vi "All-In-One_EIC-DIRC_DAQ_v2-1.vi"() -> ()   [LabVIEW 2024]
uses:
  C:/Users/hpDIRC/Desktop/eic_dirc_daq-LabVIEW_new/Thorlabs.MotionControl.Controls.dll
  Thorlabs.MotionControl.Controls.dll
  <vilib>/numeric/Random Number (Range) DBL.vi
  C:/Users/hpDIRC/Desktop/eic_dirc_daq-LabVIEW_new/Thorlabs.MotionControl.IntegratedStepperMotorsCLI.dll
  Thorlabs.MotionControl.IntegratedStepperMotorsCLI.dll
  C:/Users/hpDIRC/Desktop/eic_dirc_daq-LabVIEW_new/Thorlabs.MotionControl.Benchtop.StepperMotorCLI.dll
  Thorlabs.MotionControl.Benchtop.StepperMotorCLI.dll
  <instrlib>/Keithley 6517/Keithley 6517.lvlib
panel:
  out "NM-pts-tested":dbl caption="# Pts Tested for Alignment"
  in  "align-only":bool
  in  "run-BA":bool
  in  "run-IR":bool
  in  "PDY start":dbl=105.8
  in  "PDX start":dbl=265.0
  out "run time (min)":dbl
  out "alignment-counter":dbl=184.0 format="%#_13g"
  out "Optimized Location":dbl[](array[numeric])
  in  "Test Start Delay (s)":dbl=30.0
  out "queue-length":i32 caption="Queue Elements Remaining:"
  out "next-state-cluster-const":T1={"next-state"="", "bypass-confirm"=FALSE, "PDX"=300.0, "PDY"=150.0, "BarX"=300.0, "BarY"=150.0, "BMA"=45.0, "PDA"=85.0, "bar-note"=0, "meas#"=0}
  in  "X start":dbl=262.0
  in  "X end":dbl=263.0
  in  "Y end":dbl=121.5 format="%#_13g"
  in  "X step size":dbl=0.2 format="%#_13g"
  in  "Y step size":dbl=0.2
  in  "Y start":dbl=120.5 format="%#_13g"
  in  "centered-diode-scan":bool
  out "keep-file":bool
  out "status":string
  out "queue-size":i32
  in  "save-loc":bool
  out "stored-pos":T2 caption="Location Stored"
  out "main-stage-refs":T3
  out "state-queue":T4(array[cluster])
  in  "PDA":dbl=184.0 format="%#_13g"
  in  "BMA":dbl=45.0 format="%#_13g"
  in  "BarY":dbl=30.0 format="%#_13g"
  in  "BarX":dbl=230.0 format="%#_13g"
  in  "PDY":dbl=124.0 format="%#_13g"
  in  "PDX":dbl=274.0 format="%#_13g"
  out "bypass-confirm":bool
  out "PD Values":cluster{"PD1":dbl, "PD2":dbl, "PD3":dbl}
  out "last-PD":dbl[](array[numeric])=[1.0, 1.0, 1.0]
  in  "move-bar":bool
  out "pd_angle":dbl
  out "brewster_angle":dbl
  out "meter-visa":refnum<visa-resource-name>
  out "loop-rate":u32
  out "meter-stat":bool caption="Log Status"
  out "file-stat":bool caption="Log Status"
  out "stage-stat":bool caption="Log Status"
  out "last-save-time":string caption="Time of Last Save:"
  out "pd_y_pos":dbl
  out "pd_x_pos":dbl
  out "bar_y_pos":dbl
  out "bar_x_pos":dbl
  in  "nSamples":dbl=50.0 caption="# Samples"
  out "Current Time:":string
  in  "save-data":bool
  in  "bar-note":u16(ring) items=["Pure Beam (PB)", "Internal Reflection (IR)", "Bulk Attenuation (BA)"]
  out "pd3_v":dbl caption="PD 3" format="%#.4g"
  out "pd2_v":dbl caption="PD 2" format="%#.4g"
  out "pd1_v":dbl caption="PD 1" format="%#.4g"
  out "meter-error":errorcluster
  out "log-error":errorcluster
  out "log-path":path caption="Path Data Will Save To:"
  out "start-msg":string
  out "stage-error":errorcluster
  in  "PD Angle":refnum<k24>(container)
  in  "Brewster":refnum<k24>(container)
  in  "PD Y":refnum<k24>(container)
  in  "PD X":refnum<k24>(container)
  in  "BAR Y":refnum<k24>(container)
  in  "stop":bool
  in  "BAR X":refnum<k24>(container)
  out "pd-plt":cluster{"[0]":dbl, "[1]":dbl, "[2]":dbl}(graph) caption="Measurement History"
  # "EXPERT DEBUGGING INFO"
  # "A"
  # "A"
  # "A"
  # "Work In Progress - please do not use"
  # "Bar Note Readback:"
  # "PD ONLY SCAN - CENTERED"
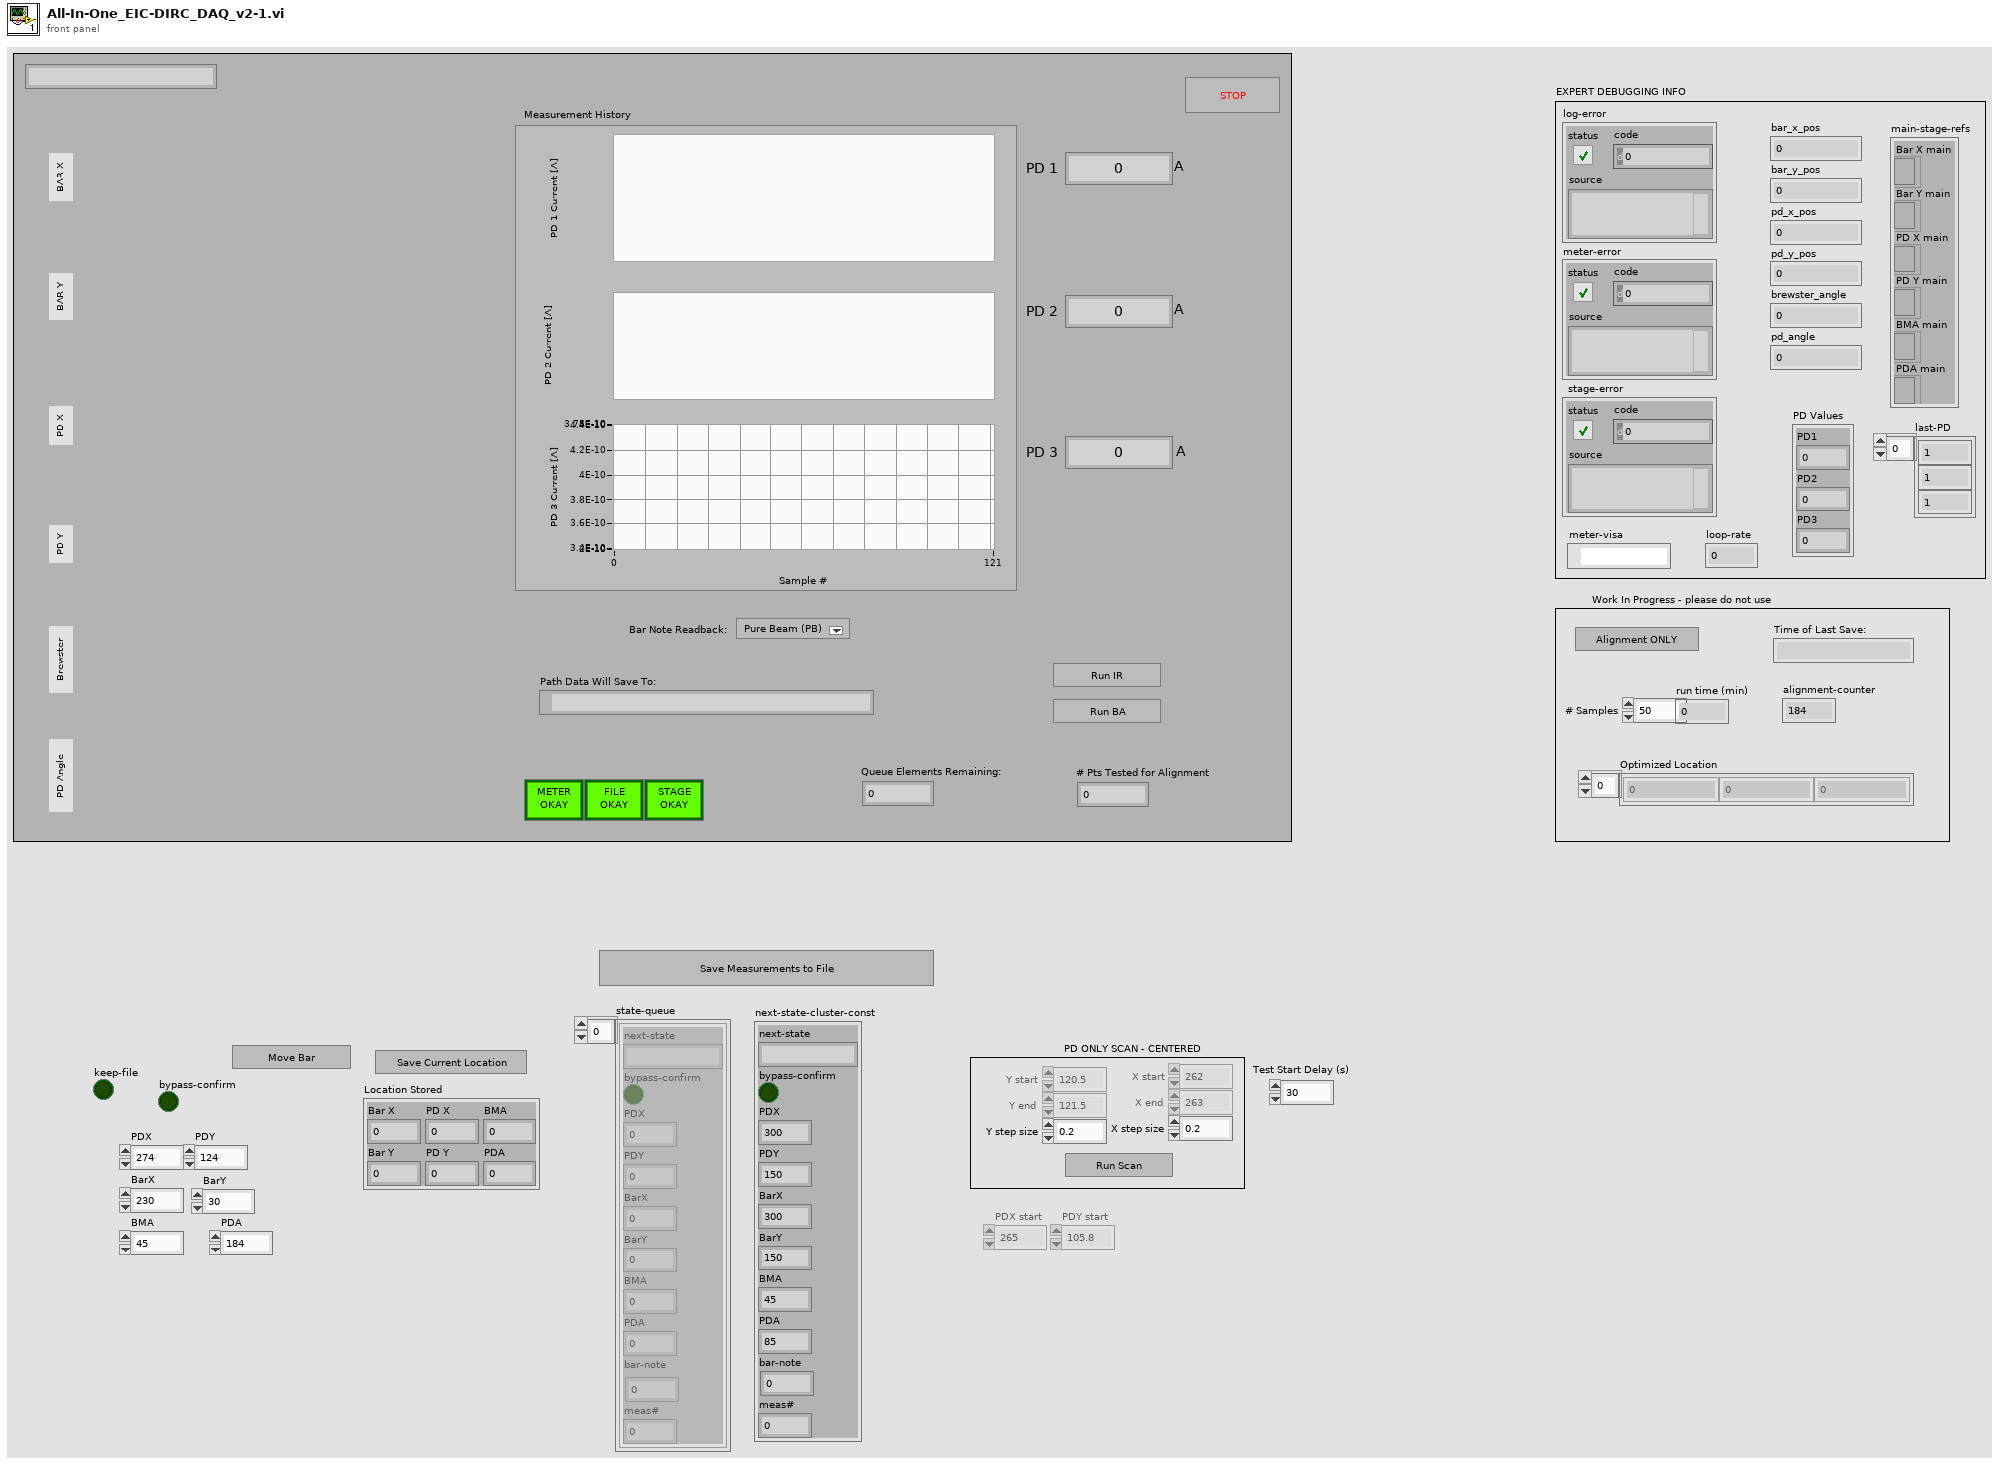
[diagram p1: front panel]
types:
  T1 = cluster{"next-state":string, "bypass-confirm":bool, "PDX":dbl, "PDY":dbl, "BarX":dbl, "BarY":dbl, "BMA":dbl, "PDA":dbl, "bar-note":u8, "meas#":u32}
  T2 = cluster{"Bar X":dbl, "Bar Y":dbl, "PD X":dbl, "PD Y":dbl, "BMA":dbl, "PDA":dbl}
  T3 = cluster{"Bar X main":refnum<k24>, "Bar Y main":refnum<k24>, "PD X main":refnum<k24>, "PD Y main":refnum<k24>, "BMA main":refnum<k24>, "PDA main":refnum<k24>}
  T4 = cluster{"next-state":string, "bypass-confirm":bool, "PDX":dbl, "PDY":dbl, "BarX":dbl, "BarY":dbl, "BMA":dbl, "PDA":dbl, "bar-note":u8, "meas#":u32}[]
  T5 = cluster{"Bar X":refnum<k24>, "Bar Y":refnum<k24>, "PD X":refnum<k24>, "PD Y":refnum<k24>, "Brewster":refnum<k24>, "PD Angle":refnum<k24>}
  T6 = enum16{"open", "replace", "create", "open or create", "replace or create", "replace or create with confirmation"}
  T7 = cluster{"alpha":dbl, "gamma":dbl, "rho":dbl, "sigma":dbl, "simplex L":dbl}
  T8 = cluster{"next-state":string, "mode-select":enum32{"IR", "Pure", "Bulk", "Bar Out", "stored-loc", "custom"}, "bypass-confirm":bool, "PDX":dbl, "PDY":dbl, "BarX":dbl, "BarY":dbl, "BMA":dbl, "PDA":dbl, "bar-note":bool}
  T9 = cluster{"error":bool, "code":i32, "source":string}
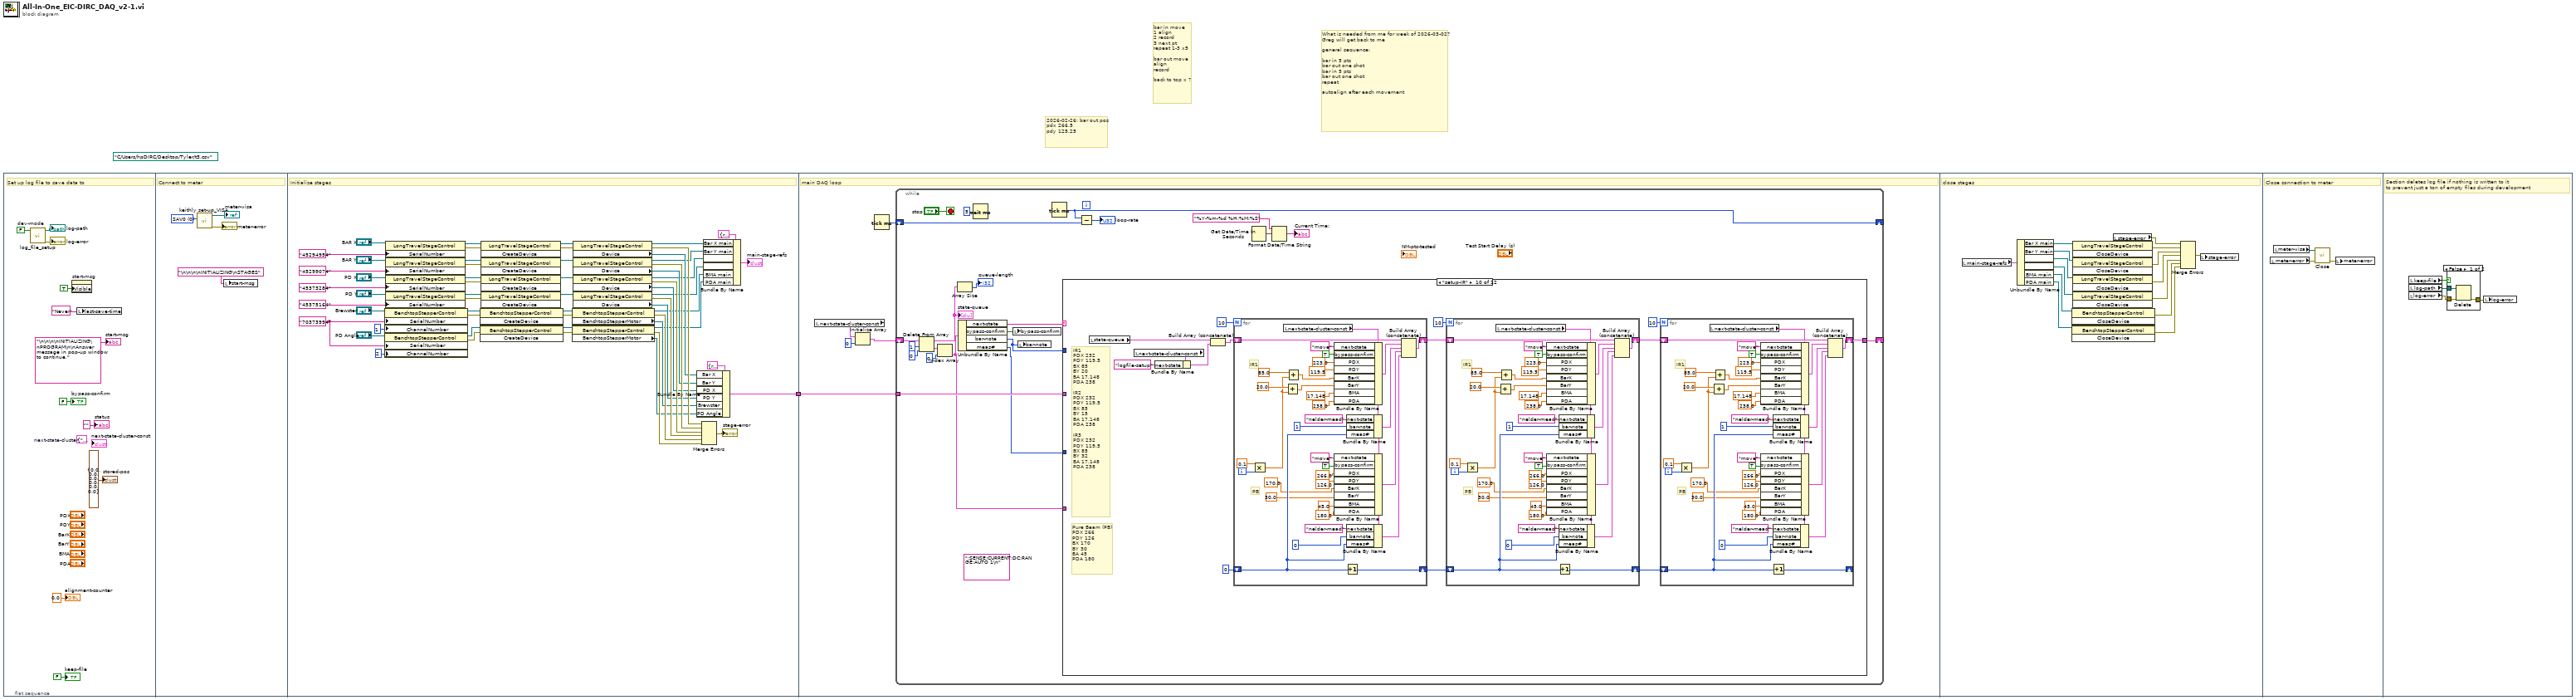
[diagram p0: block diagram]
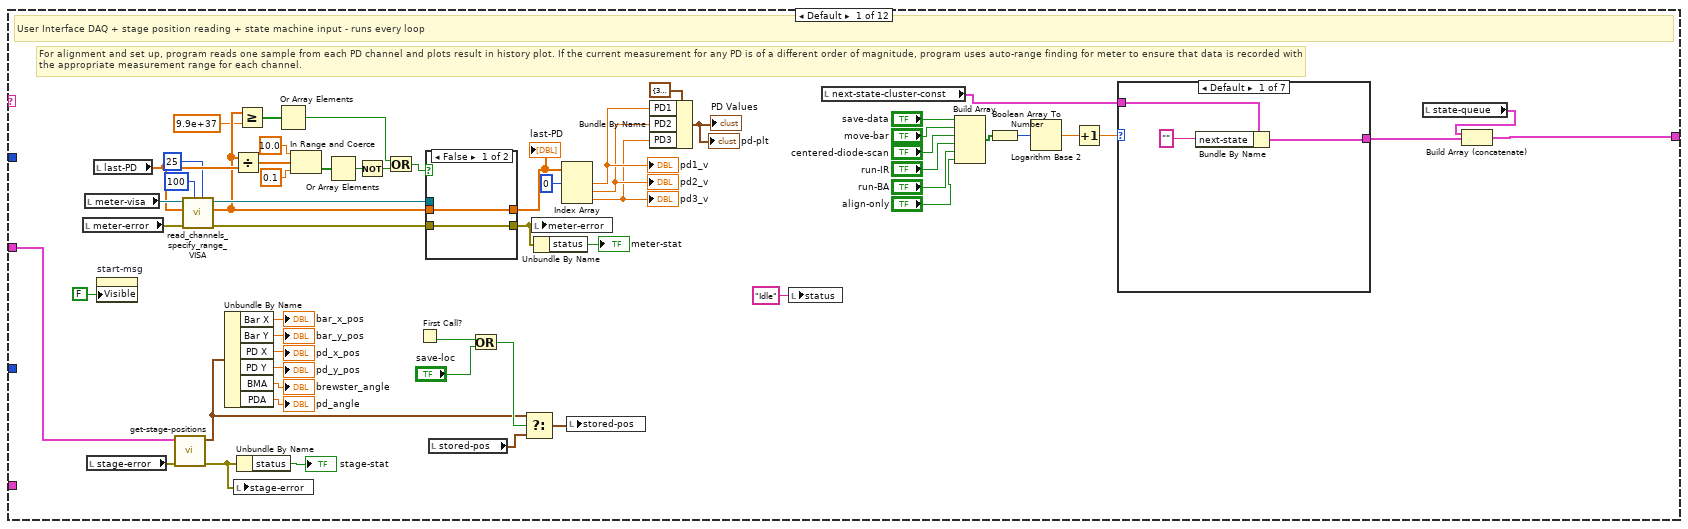
[diagram p2: hidden frame]
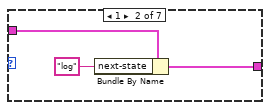
[diagram p3: hidden frame]
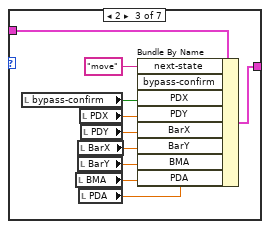
[diagram p4: hidden frame]
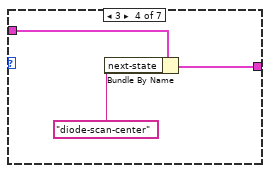
[diagram p5: hidden frame]
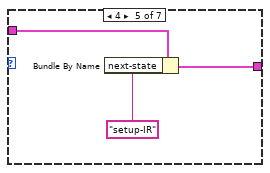
[diagram p6: hidden frame]
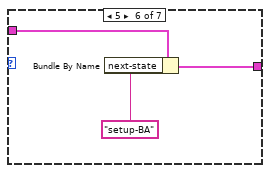
[diagram p7: hidden frame]
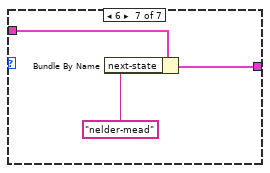
[diagram p8: hidden frame]
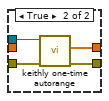
[diagram p9: hidden frame]
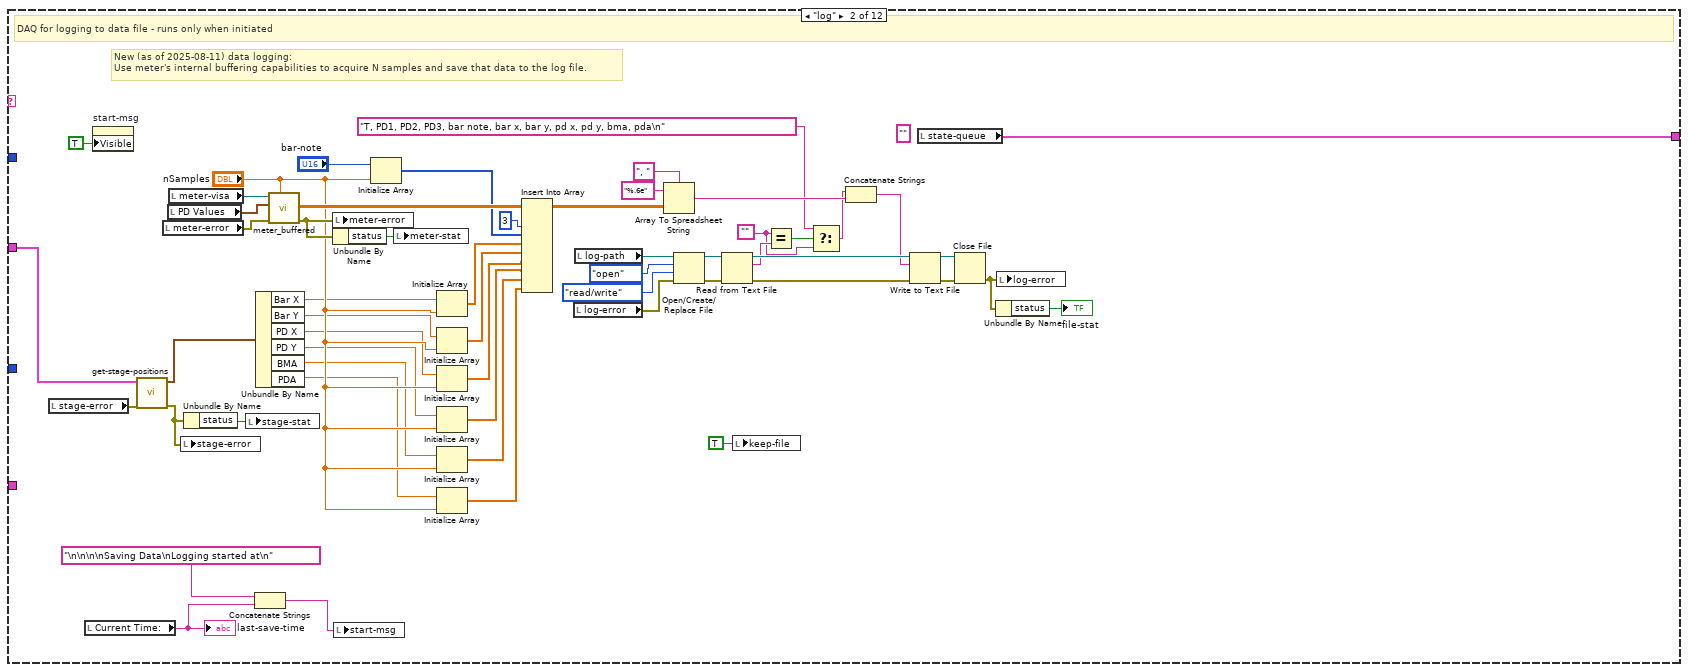
[diagram p10: hidden frame]
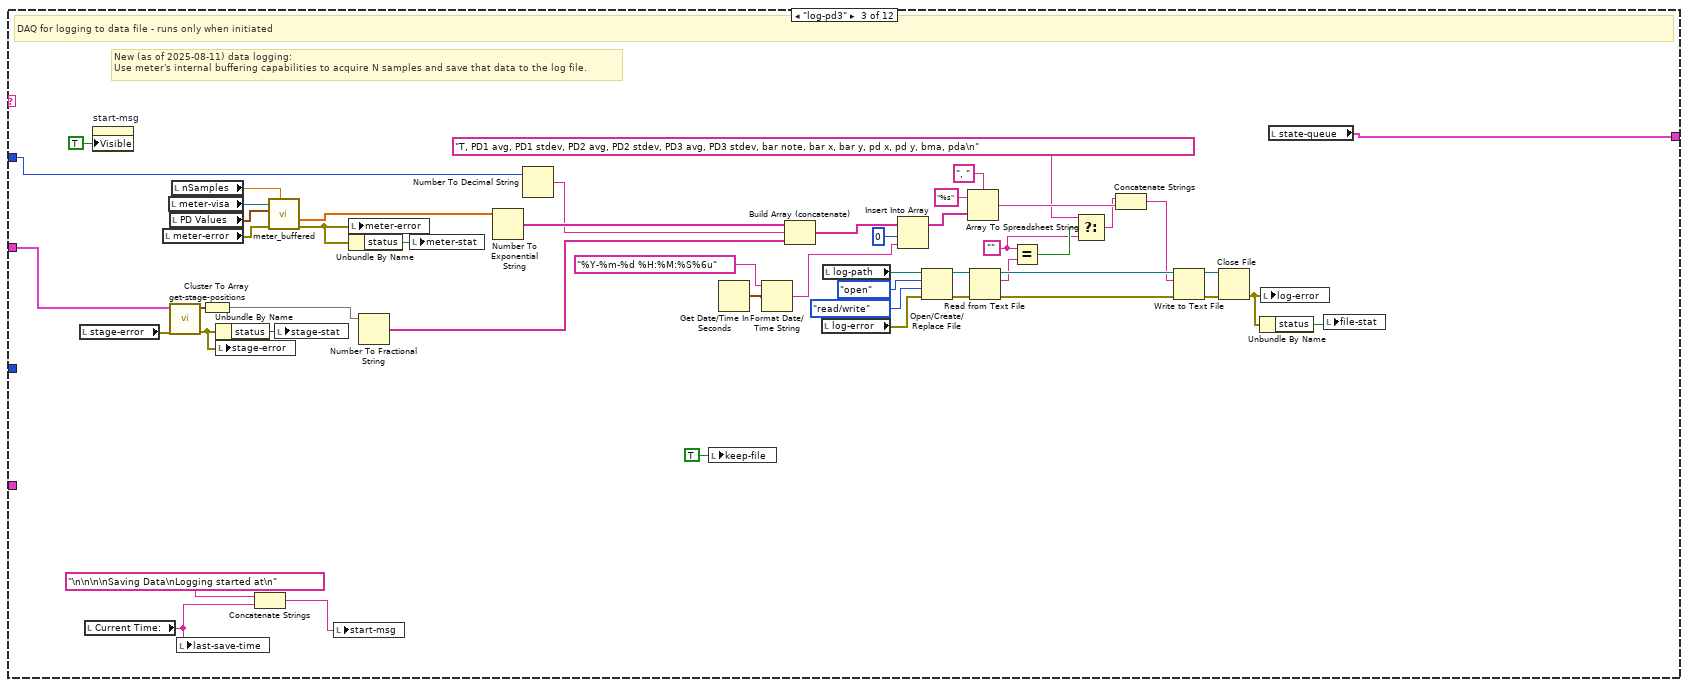
[diagram p11: hidden frame]
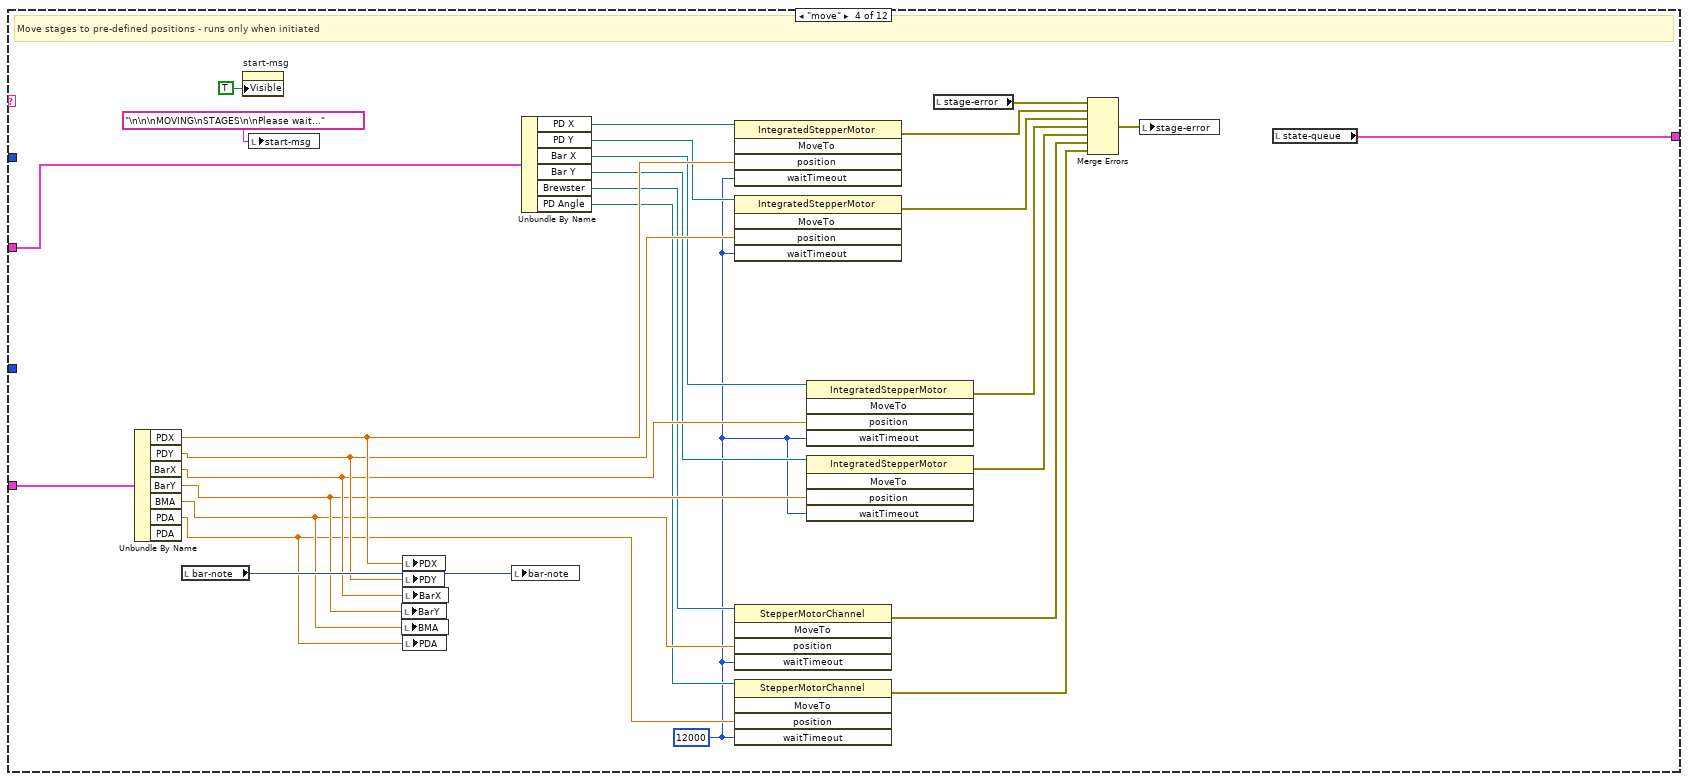
[diagram p12: hidden frame]
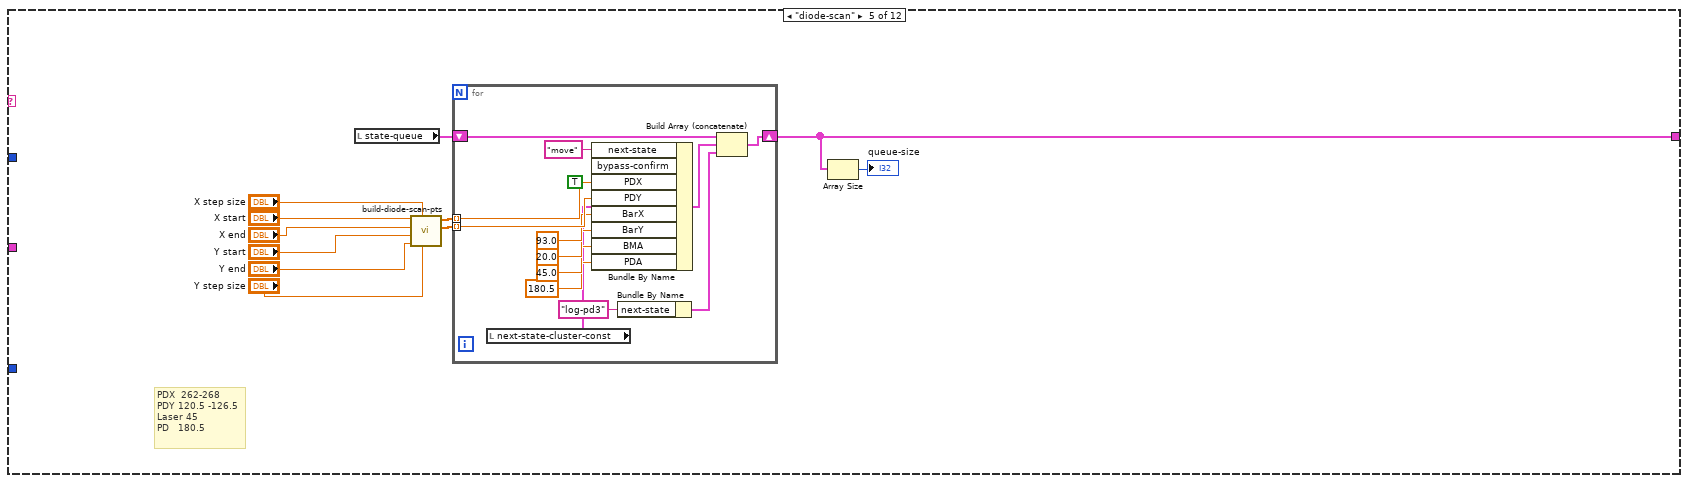
[diagram p13: hidden frame]
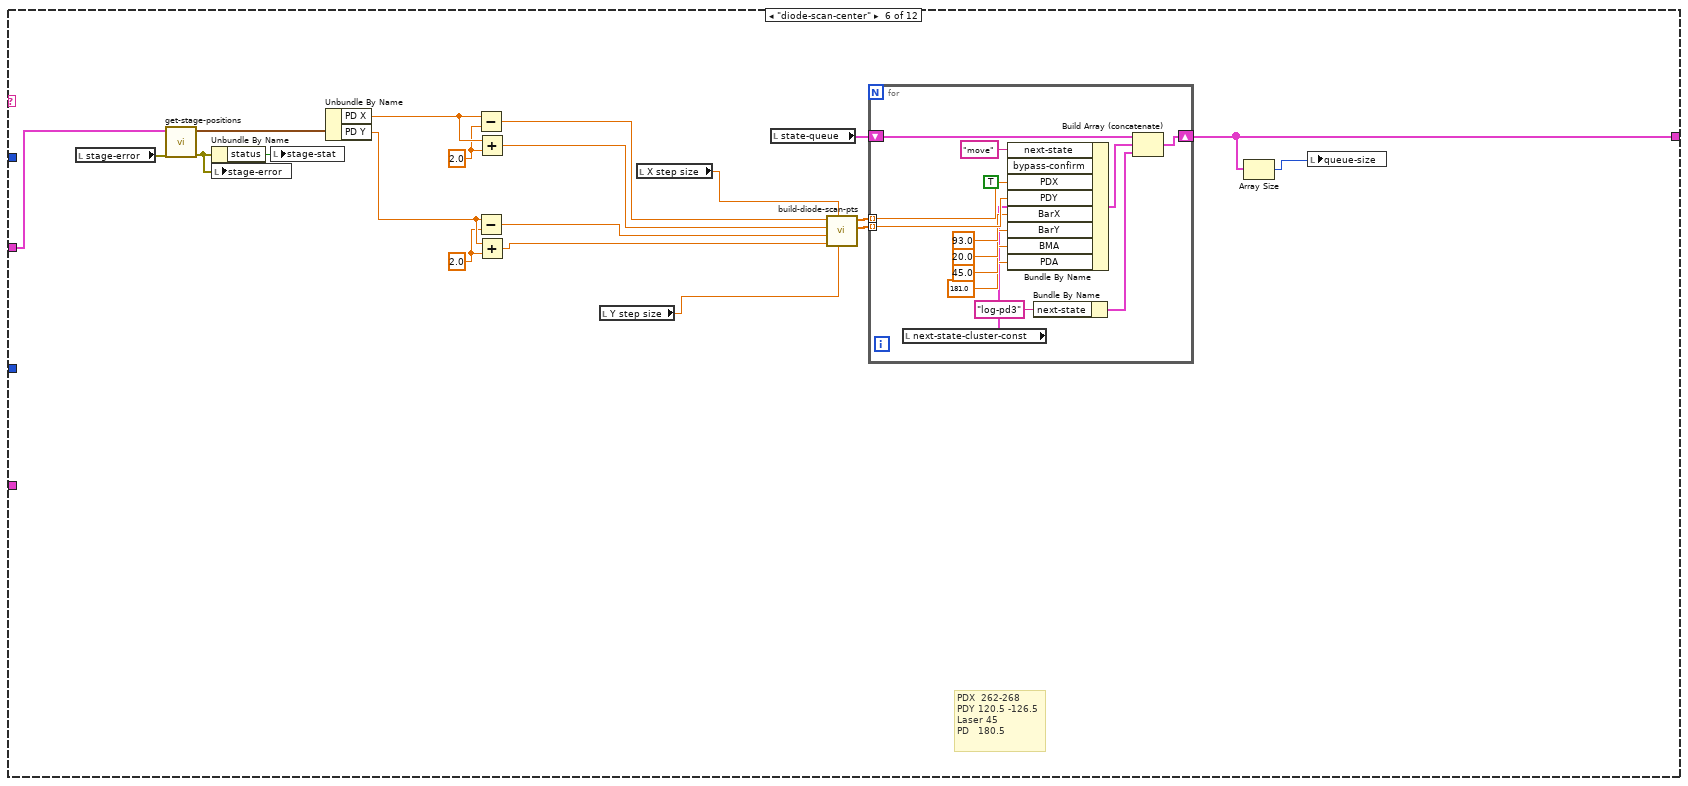
[diagram p14: hidden frame]
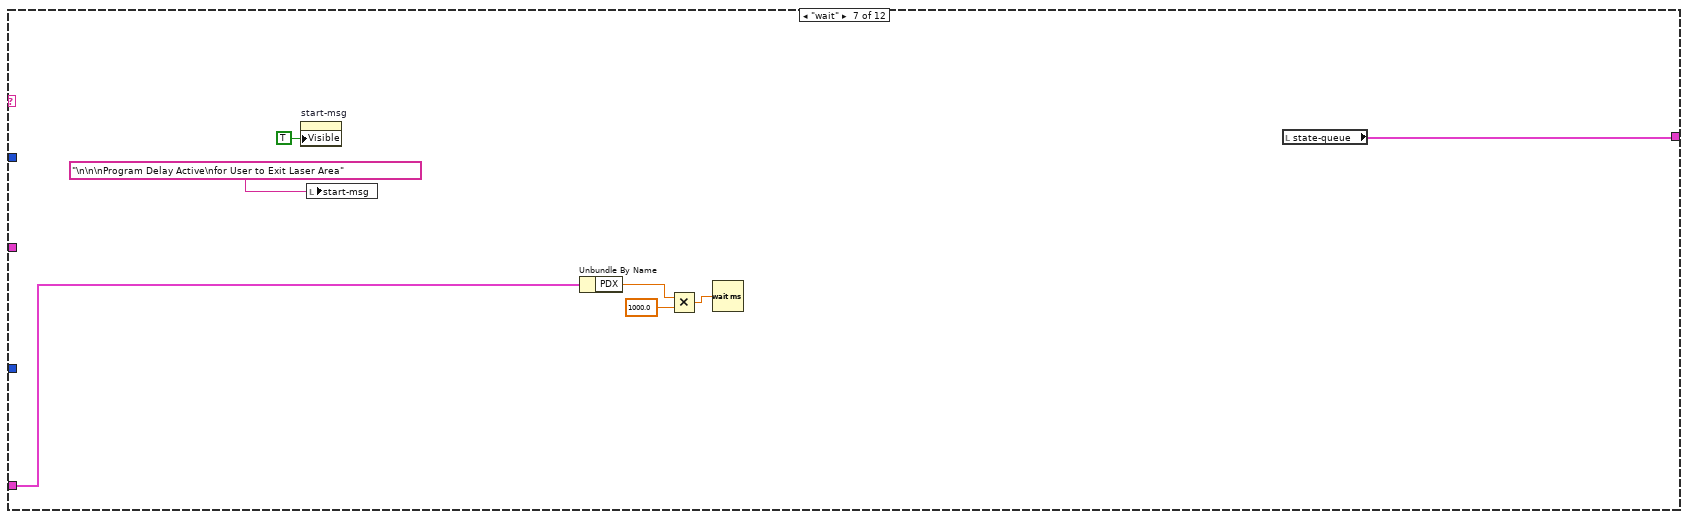
[diagram p15: hidden frame]
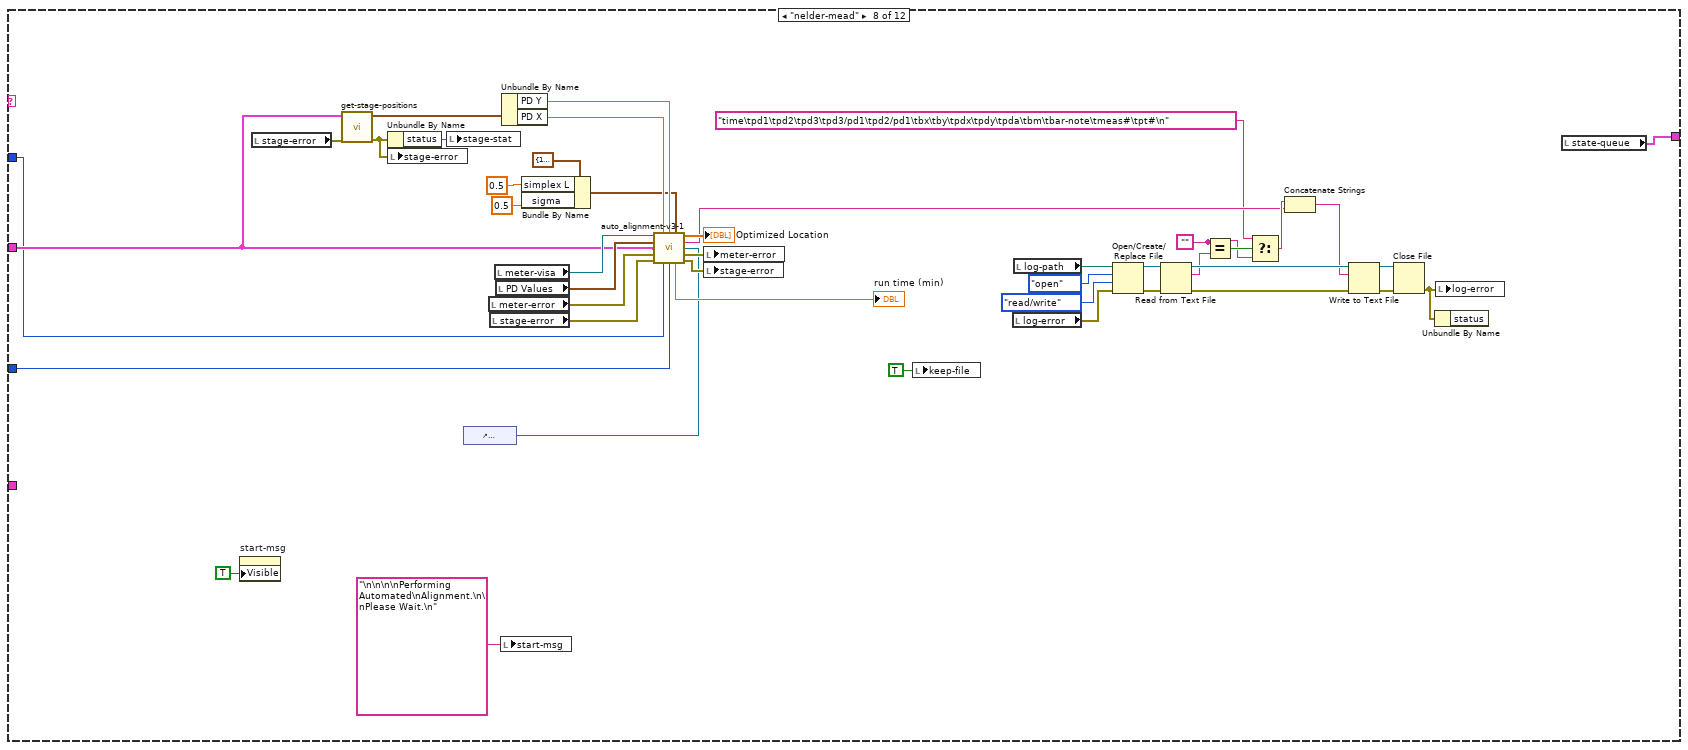
[diagram p16: hidden frame]
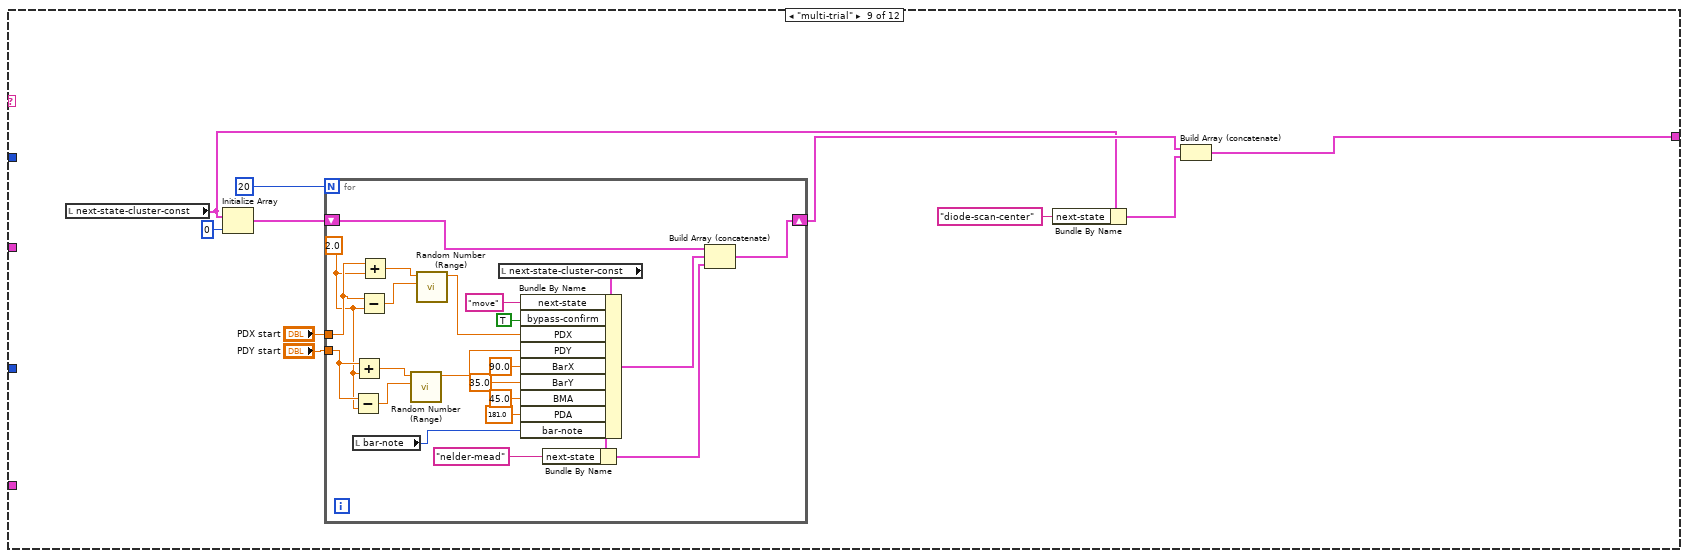
[diagram p17: hidden frame]
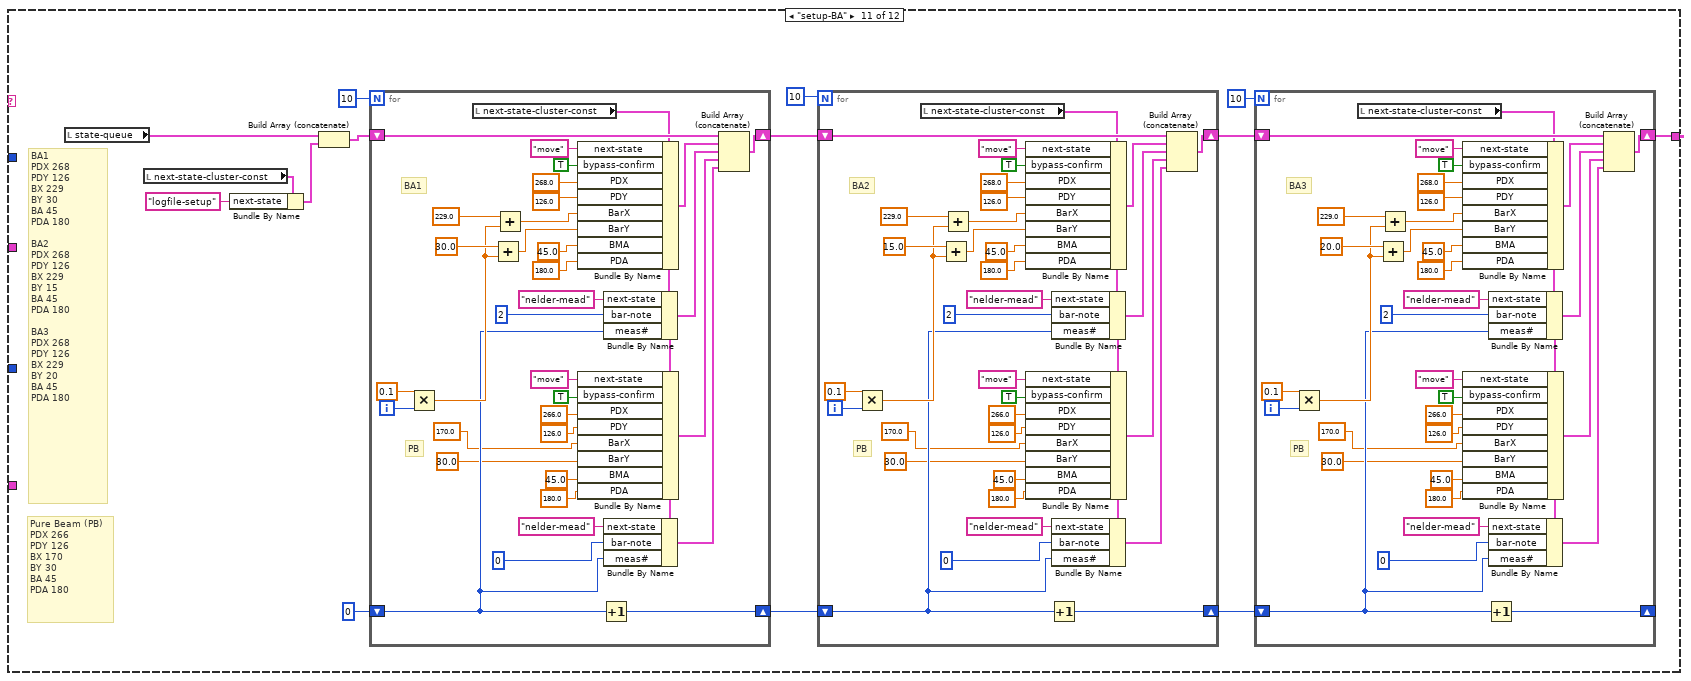
[diagram p18: hidden frame]
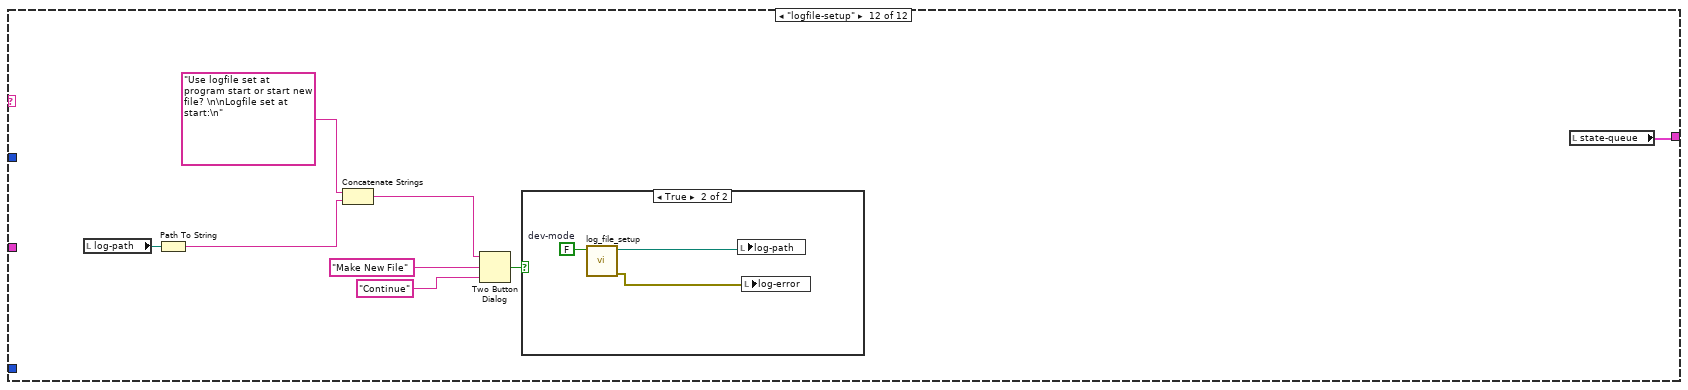
[diagram p19: hidden frame]
diagram:
  (unwired) path "C:/Users/hpDIRC/Desktop/Tyler/t3.csv" ("log-path")
  # "2026-02-26: bar out pos\npdx 266.5\npdy 125.25"
  # "bar in move\n1 align\n2 record\n3 next pt\nrepeat 1-3 x5\n\nbar out move\nalign\nrecord\n\nback to top x ?"
  # "What is needed from me for week of 2026-03-02?\nGreg will get back to me\n\ngeneral sequence:\n\nbar in 5 pts \nbar out one shot\nbar in 5 pts\nbar out one shot\nrepeat\n\nautoalign after each movement"
  n1 = flat-sequence {
    tunnel: [w25] -> w1
    tunnel: w1 -> [w77]
    frame #0 {
      w4 = FALSE  # dev-mode
      (unwired) T8 {"next-state"="", "mode-select"=enum."IR", "bypass-confirm"=FALSE, "PDX"=300.0, "PDY"=150.0, "BarX"=300.0, "BarY"=150.0, "BMA"=45.0, "PDA"=85.0, "bar-note"=FALSE}  # next-state-cluster
      # "Set up log file to save data to"
      n2 = call "log_file_setup.vi"("dev-mode"=w4) -> ("error out"=→"log-error":errorcluster, "appended path"=→"log-path":path)  [unwired: 8 in, 1 out]
      n3 = property on="start-msg" class="Str"("Visible"=TRUE) -> ()  [unwired: 2 in, 2 out]
      n4 = local write "last-save-time"("Never" ("date/time string")) -> ()
      "start-msg" <- "\n\n\n\nINITIALIZING\nPROGRAM\n\nAnswer message in pop-up window to continue." ("String")
      "bypass-confirm" <- FALSE
      "stored-pos" <- T2 {"Bar X"=0.0, "Bar Y"=0.0, "PD X"=0.0, "PD Y"=0.0, "BMA"=0.0, "PDA"=0.0} ("stage-pos")
      "status" <- "" ("status")
      "keep-file" <- FALSE
      "alignment-counter" <- 0.0 ("alignment-counter")
    }
    frame #1 {
      w13 = i16 0 items=["SAV0", "SAV1", "SAV2", "SAV3", "SAV4", "SAV5", "SAV6", "SAV7", "SAV8", "SAV9", "RST", "Preset"] ("ConfigOpt")
      # "Connect to meter"
      n5 = call "keithly set-up_VISA.vi"("ConfigOpt"=w13) -> ("error out"=→"meter-error":errorcluster, "meter-VISA"=→"meter-visa":refnum<visa-resource-name>)  [unwired: 9 in]
      n6 = local write "start-msg"("\n\n\n\nINITIALIZING\nSTAGES" ("String")) -> ()
    }
    frame #2 {
      w32 = "70373994" ("SerialNumber")
      # "Initialize stages"
      n7 = property class="BenchtopStepperControl"(reference="Brewster", "SerialNumber"=w32, "ChannelNumber"=1) -> (reference out=w58:refnum<k24>, error out=w59:errorcluster)  [unwired: 1 in]
      n8 = property class="BenchtopStepperControl"(reference="PD Angle", "SerialNumber"=w32, "ChannelNumber"=2) -> (reference out=w57:refnum<k24>, error out=w60:errorcluster)  [unwired: 1 in]
      n9 = property class="LongTravelStageControl"(reference="BAR X", "SerialNumber"="45294954") -> (reference out=w35:refnum<k24>, error out=w42:errorcluster)  [unwired: 1 in]
      n10 = property class="LongTravelStageControl"(reference="BAR Y", "SerialNumber"="45299074") -> (reference out=w36:refnum<k24>, error out=w43:errorcluster)  [unwired: 1 in]
      n11 = property class="LongTravelStageControl"(reference="PD X", "SerialNumber"="45373284") -> (reference out=w39:refnum<k24>, error out=w44:errorcluster)  [unwired: 1 in]
      n12 = property class="LongTravelStageControl"(reference="PD Y", "SerialNumber"="45375164") -> (reference out=w40:refnum<k24>, error out=w45:errorcluster)  [unwired: 1 in]
      n13 = invoke class="BenchtopStepperControl" method="CreateDevice"(reference=w58, error in=w59) -> (reference out=w55:refnum<k24>, error out=w53:errorcluster)  [unwired: 1 in, 1 out]
      n14 = invoke class="BenchtopStepperControl" method="CreateDevice"(reference=w57, error in=w60) -> (reference out=w54:refnum<k24>, error out=w56:errorcluster)  [unwired: 1 in, 1 out]
      n15 = invoke class="LongTravelStageControl" method="CreateDevice"(reference=w35, error in=w42) -> (reference out=w48:refnum<k24>, error out=w52:errorcluster)  [unwired: 1 in, 1 out]
      n16 = invoke class="LongTravelStageControl" method="CreateDevice"(reference=w36, error in=w43) -> (reference out=w49:refnum<k24>)  [unwired: 1 in, 2 out]
      n17 = invoke class="LongTravelStageControl" method="CreateDevice"(reference=w39, error in=w44) -> (reference out=w50:refnum<k24>)  [unwired: 1 in, 2 out]
      n18 = invoke class="LongTravelStageControl" method="CreateDevice"(reference=w40, error in=w45) -> (reference out=w51:refnum<k24>)  [unwired: 1 in, 2 out]
      n19 = property class="BenchtopStepperControl"(reference=w55, error in=w53) -> (reference out=w19:refnum<k24>, error out=w70:errorcluster, "BenchtopStepperMotor"=w65:refnum<k24>)
      n20 = property class="BenchtopStepperControl"(reference=w54, error in=w56) -> (reference out=w18:refnum<k24>, error out=w71:errorcluster, "BenchtopStepperMotor"=w66:refnum<k24>)
      n21 = property class="LongTravelStageControl"(reference=w48, error in=w52) -> (reference out=w23:refnum<k24>, error out=w72:errorcluster, "Device"=w61:refnum<k24>)
      n22 = property class="LongTravelStageControl"(reference=w49) -> (reference out=w22:refnum<k24>, error out=w67:errorcluster, "Device"=w62:refnum<k24>)  [unwired: 1 in]
      n23 = property class="LongTravelStageControl"(reference=w50) -> (reference out=w21:refnum<k24>, error out=w68:errorcluster, "Device"=w63:refnum<k24>)  [unwired: 1 in]
      n24 = property class="LongTravelStageControl"(reference=w51) -> (reference out=w20:refnum<k24>, error out=w69:errorcluster, "Device"=w64:refnum<k24>)  [unwired: 1 in]
      n25 = Bundle By Name(cluster=T5 {"Bar X"=refnum, "Bar Y"=refnum, "PD X"=refnum, "PD Y"=refnum, "Brewster"=refnum, "PD Angle"=refnum}, "Bar X"=w61, "Bar Y"=w62, "PD X"=w63, "PD Y"=w64, "Brewster"=w65, "PD Angle"=w66) -> (w25:T5)
      n26 = Merge Errors(w72, w67, w68, w69, w70, w71) -> (→"stage-error":errorcluster)
      n27 = Bundle By Name(cluster=T3 {"Bar X main"=refnum, "Bar Y main"=refnum, "PD X main"=refnum, "PD Y main"=refnum, "BMA main"=refnum, "PDA main"=refnum}, "Bar X main"=w23, "Bar Y main"=w22, "PD X main"=w21, "PD Y main"=w20, "BMA main"=w19, "PDA main"=w18) -> (→"main-stage-refs":T3)
    }
    frame #3 {
      # "main DAQ loop"
      n28 = local read "next-state-cluster-const"() -> (w74:T1)
      n29 = Initialize Array(w74, 0 ("dimension size")) -> (w76:T4)
      n30 = Tick Count (ms)() -> (millisecond timer value=w78:u32)
      n31 = while {
        shift-right: [w99] -> _
        shift-left: w78 -> [w98]
        tunnel: w77 -> [w96]
        shift-right: [w84] -> _
        shift-left: w76 -> [w86]
        stop <- "stop" stop-if-true
        (unwired) ":SENSE:CURRENT:DC:RANGE:AUTO 1\n"
        n32 = Delete From Array(array=w86, length=1, index=0) -> (deleted portion=w85:T4, array with subset deleted=w82:T4)
        "state-queue" <- w82
        n33 = Index Array(array=w85, index=0) -> (element=w83:T1)
        n34 = Array Size(array=w82) -> (size(s)=→"queue-length":i32)
        n35 = Unbundle By Name(w83) -> ("next-state"=w88:string, "bypass-confirm"=w87:bool, "bar-note"=w81:u8, "meas#"=w80:u32)
        n36 = Wait (ms)(milliseconds to wait=u32 5) -> ()  [unwired: 1 out]
        n37 = local write "bypass-confirm"(w87) -> ()
        n38 = local write "bar-note"(w81) -> ()
        n39 = Tick Count (ms)() -> (millisecond timer value=w99:u32)
        n40 = case shown="\"setup-IR\"" w88 {
          tunnel: w96 -> [w151 w212 w277 w324 _ w359 _ w414 _ _ _ _]
          tunnel: [w123 w223 w282 w323 w333 w367 w387 w435 w438 w472 w588 w707] -> w84
          tunnel: w83 -> [_ _ _ w320 _ _ w388 _ _ _ _ _]
          tunnel: w81 -> [_ _ w260 _ _ _ _ w413 _ _ _ _]
          tunnel: w80 -> [_ _ _ _ _ _ _ w412 _ _ _ _]
          frame Default {
            # "For alignment and set up, program reads one sample from each PD channel and plots result in history plot. If the current measurement for any PD is of a different order of magnitude, program uses auto-range finding for meter to ensure that data is recorded with the appropriate measurement range for each channel."
            # "User Interface DAQ + stage position reading + state machine input - runs every loop"
            n41 = local read "meter-error"() -> (w148:errorcluster)
            n42 = local read "meter-visa"() -> (w149:refnum<visa-resource-name>)
            n43 = local read "stage-error"() -> (w150:errorcluster)
            n44 = local read "last-PD"() -> (w139:dbl[])
            n45 = property on="start-msg" class="Str"("Visible"=FALSE) -> ()  [unwired: 2 in, 2 out]
            n46 = call "get-stage-positions.vi"("error in (no error)"=w150, "Cluster"=w151) -> ("error out"=w136:errorcluster, "stage positions"=w109:T2)  [unwired: 8 in]
            n47 = call "read_channels_specify_range_VISA.vi"("postDAQ  wait ms"=u32 25, "preDAQ  wait ms"=u32 100, "error in"=w148, "range"=w139, "VISA resource in"=w149) -> ("error out"=w141:T9, "data"=w129:dbl[], "VISA resource out"=w140:refnum<visa-resource-name>)  [unwired: 4 in]
            n48 = Unbundle By Name(w109) -> ("Bar X"=→"bar_x_pos":dbl, "Bar Y"=→"bar_y_pos":dbl, "PD X"=→"pd_x_pos":dbl, "PD Y"=→"pd_y_pos":dbl, "BMA"=→"brewster_angle":dbl, "PDA"=→"pd_angle":dbl)
            n49 = Divide(x=w129, y=w139) -> (x/y=w144:dbl[])
            n50 = local write "stage-error"(w136) -> ()
            n51 = Greater Or Equal?(x=w129, y=9.9e+37) -> (x >= y?=w127:bool[])
            n52 = Unbundle By Name(w136) -> ("status"=→"stage-stat":bool)
            n53 = Or Array Elements(Boolean array=w127) -> (logical OR=w126:bool)
            n54 = In Range and Coerce(upper limit=10.0, x=w144, lower limit=0.1) -> (In Range?=w142:bool[])  [unwired: 1 out]
            n55 = Or Array Elements(Boolean array=w142) -> (logical OR=w143:bool)
            n56 = Not(x=w143) -> (.not. x?=w131:bool)
            n57 = Or(x=w126, y=w131) -> (x .or. y?=w130:bool)
            n58 = First Call?() -> (First Call?: T/F=w119:bool)
            n59 = case shown="False" w130 {
              tunnel: w141 -> [w189 w193]
              tunnel: [w189 w192] -> w157
              tunnel: [w188 w191] -> w152
              tunnel: w129 -> [w188 _]
              tunnel: w140 -> [_ w190]
              frame False {
              }
              frame True {
                n60 = call "keithly one-time autorange.vi"("error in"=w193, "VISA in"=w190) -> ("error out"=w192:errorcluster, "data"=w191:dbl[])  [unwired: 7 in, 1 out]
              }
            }
            "last-PD" <- w152
            n61 = local read "stored-pos"() -> (w120:T2)
            n62 = Or(x=w119, y="save-loc") -> (x .or. y?=w117:bool)
            n63 = Select(t=w109, s=w117, f=w120) -> (s? t:f=w121:T2)
            n64 = local write "meter-error"(w157) -> ()
            n65 = Unbundle By Name(w157) -> ("status"=→"meter-stat":bool)
            n66 = Index Array(array=w152, index #1=0 ("index")) -> (element #1=w155:dbl, element #2=w154:dbl, element #3=w153:dbl)  [unwired: 2 in]
            "pd3_v" <- w153
            "pd2_v" <- w154
            "pd1_v" <- w155
            n67 = local write "stored-pos"(w121) -> ()
            n68 = Bundle By Name(cluster=cluster{"PD1":dbl, "PD2":dbl, "PD3":dbl} {"PD1"=3e-05, "PD2"=3e-05, "PD3"=3e-05} ("PD ranges"), "PD1"=w155, "PD2"=w154, "PD3"=w153) -> (→"pd-plt" →"PD Values":cluster{"PD1":dbl, "PD2":dbl, "PD3":dbl})
            n69 = local write "status"("Idle" ("status")) -> ()
            n70 = local read "next-state-cluster-const"() -> (w107:T1)
            n71 = Build Array("save-data", "move-bar", "centered-diode-scan", "run-IR", "run-BA", "align-only") -> (w133:bool[])
            n72 = Boolean Array To Number(Boolean array=w133) -> (number=w104:u32)
            n73 = Logarithm Base 2(1:w104) -> (0:w106:dbl)
            n74 = Increment(x=w106) -> (x+1=w105:dbl)
            n75 = case shown="Default" w105 {
              tunnel: w107 -> [w162 w165 w175 w178 w181 w184 w187]
              tunnel: [w160 w163 w173 w176 w179 w182 w185] -> w122
              frame Default {
                n76 = Bundle By Name(cluster=w162, "next-state"="") -> (w160:T1)
              }
              frame 1 {
                n77 = Bundle By Name(cluster=w165, "next-state"="log") -> (w163:T1)
              }
              frame 2 {
                n78 = local read "bypass-confirm"() -> (w166:bool)
                n79 = local read "BMA"() -> (w171:dbl)
                n80 = local read "BarX"() -> (w169:dbl)
                n81 = local read "BarY"() -> (w170:dbl)
                n82 = local read "PDA"() -> (w172:dbl)
                n83 = local read "PDX"() -> (w167:dbl)
                n84 = local read "PDY"() -> (w168:dbl)
                n85 = Bundle By Name(cluster=w175, "next-state"="move", "bypass-confirm"=w166, "PDX"=w167, "PDY"=w168, "BarX"=w169, "BarY"=w170, "BMA"=w171, "PDA"=w172) -> (w173:T1)
              }
              frame 3 {
                n86 = Bundle By Name(cluster=w178, "next-state"="diode-scan-center") -> (w176:T1)
              }
              frame 4 {
                n87 = Bundle By Name(cluster=w181, "next-state"="setup-IR") -> (w179:T1)
              }
              frame 5 {
                n88 = Bundle By Name(cluster=w184, "next-state"="setup-BA") -> (w182:T1)
              }
              frame 6 {
                n89 = Bundle By Name(cluster=w187, "next-state"="nelder-mead") -> (w185:T1)
              }
            }
            n90 = local read "state-queue"() -> (w124:T4)
            n91 = Build Array (concatenate)(w124, w122) -> (w123:T4)
          }
          frame "log" {
            w198 = ""
            (unwired) ""
            # "New (as of 2025-08-11) data logging:\nUse meter's internal buffering capabilities to acquire N samples and save that data to the log file."
            # "DAQ for logging to data file - runs only when initiated"
            n92 = local read "stage-error"() -> (w211:errorcluster)
            n93 = local read "Current Time:"() -> (w221:string)
            "last-save-time" <- w221
            n94 = property on="start-msg" class="Str"("Visible"=TRUE) -> ()  [unwired: 2 in, 2 out]
            n95 = call "get-stage-positions.vi"("error in (no error)"=w211, "Cluster"=w212) -> ("error out"=w210:errorcluster, "stage positions"=w208:T2)  [unwired: 8 in]
            n96 = local read "meter-error"() -> (w247:errorcluster)
            n97 = local read "PD Values"() -> (w226:cluster{"PD1":dbl, "PD2":dbl, "PD3":dbl})
            n98 = local read "meter-visa"() -> (w248:refnum<visa-resource-name>)
            n99 = local write "stage-error"(w210) -> ()
            n100 = Unbundle By Name(w210) -> ("status"=w209:bool)
            n101 = local write "stage-stat"(w209) -> ()
            n102 = Concatenate Strings("\n\n\n\nSaving Data\nLogging started at\n" ("String"), w221) -> (w224:string)
            n103 = Unbundle By Name(w208) -> ("Bar X"=w207:dbl, "Bar Y"=w206:dbl, "PD X"=w205:dbl, "PD Y"=w204:dbl, "BMA"=w203:dbl, "PDA"=w202:dbl)
            n104 = call "meter_buffered.vi"("Samples"="nSamples", "error in"=w247, "PD ranges"=w226, "meter-VISA"=w248) -> ("error out"=w227:errorcluster, "ch1-3 data"=w235:dbl[][])  [unwired: 3 in, 3 out]
            n105 = local write "meter-error"(w227) -> ()
            n106 = Unbundle By Name(w227) -> ("status"=w228:bool)
            n107 = local write "start-msg"(w224) -> ()
            n108 = Initialize Array("bar-note", "nSamples") -> (w233:u16[])
            n109 = local write "meter-stat"(w228) -> ()
            n110 = Initialize Array(w207, "nSamples") -> (w218:dbl[])
            n111 = Initialize Array(w206, "nSamples") -> (w217:dbl[])
            n112 = Initialize Array(w205, "nSamples") -> (w216:dbl[])
            n113 = Initialize Array(w204, "nSamples") -> (w215:dbl[])
            n114 = Initialize Array(w203, "nSamples") -> (w214:dbl[])
            n115 = Initialize Array(w202, "nSamples") -> (w213:dbl[])
            n116 = Insert Into Array(array=w235, index (col)=3 ("disabled index (col)"), new element #1=w233, new element #2=w218, new element #3=w217, new element #4=w216, new element #5=w215, new element #6=w214, new element #7=w213) -> (w220:dbl[][])  [unwired: 1 in]
            n117 = local read "log-error"() -> (w245:errorcluster)
            n118 = local read "log-path"() -> (w246:path)
            n119 = Array To Spreadsheet String(delimiter (Tab)=", ", array=w220, 3:"%.6e" ("format string")) -> (spreadsheet string=w230:string)
            n120 = Open/Create/Replace File(file path (use dialog)=w246, error in=w245, operation (0:open)=T6."open", access (0:read/write)=enum16{"read/write", "read-only", "write-only"}."read/write") -> (refnum out=w244:refnum<file>, error out=w240:errorcluster)  [unwired: 2 in, 1 out]
            n121 = Read from Text File(file (use dialog)=w244, error in=w240) -> (refnum out=w241:refnum<file>, text=w200:string, error out=w239:errorcluster)  [unwired: 2 in, 1 out]
            n122 = local write "keep-file"(TRUE ("keep-file")) -> ()
            n123 = Equal?(x=w198, y=w200) -> (x = y?=w199:bool)
            n124 = Select(t="T, PD1, PD2, PD3, bar note, bar x, bar y, pd x, pd y, bma, pda\n", s=w199, f=w198) -> (s? t:f=w195:string)
            n125 = Concatenate Strings(w195, w230) -> (w196:string)
            n126 = Write to Text File(file (use dialog)=w241, text=w196, error in=w239) -> (refnum out=w243:refnum<file>, error out=w242:errorcluster)  [unwired: 1 in, 1 out]
            n127 = local read "state-queue"() -> (w223:T4)
            n128 = Close File(refnum=w243, error in=w242) -> (error out=w238:errorcluster)  [unwired: 1 out]
            n129 = Unbundle By Name(w238) -> ("status"=→"file-stat":bool)
            n130 = local write "log-error"(w238) -> ()
          }
          frame "log-pd3" {
            w262 = ""
            # "New (as of 2025-08-11) data logging:\nUse meter's internal buffering capabilities to acquire N samples and save that data to the log file."
            # "DAQ for logging to data file - runs only when initiated"
            n131 = local read "stage-error"() -> (w276:errorcluster)
            n132 = local read "Current Time:"() -> (w280:string)
            n133 = property on="start-msg" class="Str"("Visible"=TRUE) -> ()  [unwired: 2 in, 2 out]
            n134 = local read "meter-error"() -> (w250:errorcluster)
            n135 = local read "meter-visa"() -> (w252:refnum<visa-resource-name>)
            n136 = local read "PD Values"() -> (w251:cluster{"PD1":dbl, "PD2":dbl, "PD3":dbl})
            n137 = call "get-stage-positions.vi"("error in (no error)"=w276, "Cluster"=w277) -> ("error out"=w275:errorcluster, "stage positions"=w274:T2)  [unwired: 8 in]
            n138 = local read "nSamples"() -> (w253:dbl)
            n139 = local write "last-save-time"(w280) -> ()
            n140 = Cluster To Array(cluster=w274) -> (array=w259:dbl[])
            n141 = Unbundle By Name(w275) -> ("status"=w278:bool)
            n142 = local write "stage-error"(w275) -> ()
            n143 = Concatenate Strings("\n\n\n\nSaving Data\nLogging started at\n" ("String"), w280) -> (w283:string)
            n144 = call "meter_buffered.vi"("Samples"=w253, "error in"=w250, "PD ranges"=w251, "meter-VISA"=w252) -> ("error out"=w254:errorcluster, "stats-out"=w249:dbl[])  [unwired: 3 in, 3 out]
            n145 = local write "stage-stat"(w278) -> ()
            n146 = local write "start-msg"(w283) -> ()
            n147 = local write "meter-error"(w254) -> ()
            n148 = Unbundle By Name(w254) -> ("status"=w285:bool)
            n149 = Number To Fractional String(number=w259) -> (F-format string=w255:string[])  [unwired: 3 in]
            n150 = local write "meter-stat"(w285) -> ()
            n151 = Number To Exponential String(number=w249) -> (E-format string=w258:string[])  [unwired: 3 in]
            n152 = Number To Decimal String(number=w260) -> (decimal integer string=w256:string)  [unwired: 1 in]
            n153 = local write "keep-file"(TRUE ("keep-file")) -> ()
            n154 = Get Date/Time In Seconds() -> (seconds since 1Jan1904=w273:timestamp)
            n155 = Format Date/Time String(time format string (%c)="%Y-%m-%d %H:%M:%S%6u", seconds (now)=w273) -> (date/time string=w269:string)  [unwired: 1 in]
            n156 = Build Array (concatenate)(w258, w256, w255) -> (w257:string[])
            n157 = local read "log-error"() -> (w297:errorcluster)
            n158 = local read "log-path"() -> (w298:path)
            n159 = Insert Into Array(array=w257, index=0, new element=w269) -> (w270:string[])
            n160 = Open/Create/Replace File(file path (use dialog)=w298, error in=w297, operation (0:open)=T6."open", access (0:read/write)=enum16{"read/write", "read-only", "write-only"}."read/write") -> (refnum out=w296:refnum<file>, error out=w292:errorcluster)  [unwired: 2 in, 1 out]
            n161 = Array To Spreadsheet String(delimiter (Tab)=", ", array=w270, 3:"%s" ("format string")) -> (spreadsheet string=w286:string)
            n162 = Read from Text File(file (use dialog)=w296, error in=w292) -> (refnum out=w293:refnum<file>, text=w266:string, error out=w291:errorcluster)  [unwired: 2 in, 1 out]
            n163 = Equal?(x=w262, y=w266) -> (x = y?=w263:bool)
            n164 = Select(t="T, PD1 avg, PD1 stdev, PD2 avg, PD2 stdev, PD3 avg, PD3 stdev, bar note, bar x, bar y, pd x, pd y, bma, pda\n", s=w263, f=w262) -> (s? t:f=w264:string)
            n165 = Concatenate Strings(w264, w286) -> (w265:string)
            n166 = Write to Text File(file (use dialog)=w293, text=w265, error in=w291) -> (refnum out=w295:refnum<file>, error out=w294:errorcluster)  [unwired: 1 in, 1 out]
            n167 = Close File(refnum=w295, error in=w294) -> (error out=w290:errorcluster)  [unwired: 1 out]
            n168 = Unbundle By Name(w290) -> ("status"=w279:bool)
            n169 = local write "log-error"(w290) -> ()
            n170 = local read "state-queue"() -> (w282:T4)
            n171 = local write "file-stat"(w279) -> ()
          }
          frame "move" {
            w299 = 12000 ("waitTimeout")
            # "Move stages to pre-defined positions - runs only when initiated"
            n172 = Unbundle By Name(w320) -> ("PDX"=w319:dbl, "PDY"=w318:dbl, "BarX"=w317:dbl, "BarY"=w316:dbl, "BMA"=w315:dbl, "PDA"=w314:dbl)  [unwired: 1 out]
            n173 = local read "bar-note"() -> (w325:u16)
            n174 = property on="start-msg" class="Str"("Visible"=TRUE) -> ()  [unwired: 2 in, 2 out]
            n175 = local write "start-msg"("\n\n\nMOVING\nSTAGES\n\nPlease wait..." ("String")) -> ()
            n176 = local write "BarY"(w316) -> ()
            n177 = local write "BMA"(w315) -> ()
            n178 = local write "PDX"(w319) -> ()
            n179 = local write "PDY"(w318) -> ()
            n180 = local write "BarX"(w317) -> ()
            n181 = local write "PDA"(w314) -> ()
            n182 = local write "bar-note"(w325) -> ()
            n183 = Unbundle By Name(w324) -> ("PD X"=w305:refnum<k24>, "PD Y"=w300:refnum<k24>, "Bar X"=w301:refnum<k24>, "Bar Y"=w302:refnum<k24>, "Brewster"=w303:refnum<k24>, "PD Angle"=w304:refnum<k24>)
            n184 = invoke class="IntegratedStepperMotor" method="MoveTo"(reference=w305, "position"=w319, "waitTimeout"=w299) -> (error out=w312:errorcluster)  [unwired: 2 in, 4 out]
            n185 = invoke class="IntegratedStepperMotor" method="MoveTo"(reference=w300, "position"=w318, "waitTimeout"=w299) -> (error out=w311:errorcluster)  [unwired: 2 in, 4 out]
            n186 = invoke class="StepperMotorChannel" method="MoveTo"(reference=w303, "position"=w315, "waitTimeout"=w299) -> (error out=w308:errorcluster)  [unwired: 2 in, 4 out]
            n187 = invoke class="StepperMotorChannel" method="MoveTo"(reference=w304, "position"=w314, "waitTimeout"=w299) -> (error out=w307:errorcluster)  [unwired: 2 in, 4 out]
            n188 = invoke class="IntegratedStepperMotor" method="MoveTo"(reference=w301, "position"=w317, "waitTimeout"=w299) -> (error out=w310:errorcluster)  [unwired: 2 in, 4 out]
            n189 = invoke class="IntegratedStepperMotor" method="MoveTo"(reference=w302, "position"=w316, "waitTimeout"=w299) -> (error out=w309:errorcluster)  [unwired: 2 in, 4 out]
            n190 = local read "stage-error"() -> (w313:errorcluster)
            n191 = Merge Errors(w313, w312, w311, w310, w309, w308, w307) -> (w306:errorcluster)
            n192 = local write "stage-error"(w306) -> ()
            n193 = local read "state-queue"() -> (w323:T4)
          }
          frame "diode-scan" {
            # "PDX  262-268\nPDY 120.5 -126.5\nLaser 45\nPD   180.5"
            n194 = local read "state-queue"() -> (w336:T4)
            n195 = call "build-diode-scan-pts.vi"("Y step size"="Y step size", "X step size"="X step size", "Y end"="Y end", "Y start"="Y start", "X end"="X end", "X start"="X start") -> ("y"=w334:dbl[], "x"=w335:dbl[])  [unwired: 4 in]
            n196 = for {
              tunnel: w335 -> [w350] mode=indexing
              tunnel: w334 -> [w349] mode=indexing
              shift-right: [w343] -> w333
              shift-left: w336 -> [w345]
              n197 = local read "next-state-cluster-const"() -> (w337:T1)
              n198 = Bundle By Name(cluster=w337, "next-state"="move", "bypass-confirm"=TRUE, "PDX"=w350, "PDY"=w349, "BarX"=93.0, "BarY"=20.0, "BMA"=45.0, "PDA"=180.5) -> (w344:T1)
              n199 = Bundle By Name(cluster=w337, "next-state"="log-pd3") -> (w338:T1)
              n200 = Build Array (concatenate)(w345, w344, w338) -> (w343:T4)
            }
            n201 = Array Size(array=w333) -> (size(s)=→"queue-size":i32)
          }
          frame "diode-scan-center" {
            w354 = 2.0 ("y")
            w353 = 2.0 ("y")
            # "PDX  262-268\nPDY 120.5 -126.5\nLaser 45\nPD   180.5"
            n202 = local read "stage-error"() -> (w362:errorcluster)
            n203 = call "get-stage-positions.vi"("error in (no error)"=w362, "Cluster"=w359) -> ("error out"=w361:errorcluster, "stage positions"=w360:T2)  [unwired: 8 in]
            n204 = Unbundle By Name(w361) -> ("status"=w363:bool)
            n205 = local write "stage-error"(w361) -> ()
            n206 = local write "stage-stat"(w363) -> ()
            n207 = Unbundle By Name(w360) -> ("PD X"=w358:dbl, "PD Y"=w355:dbl)
            n208 = Subtract(x=w358, y=w353) -> (x-y=w357:dbl)
            n209 = Subtract(x=w355, y=w354) -> (x-y=w352:dbl)
            n210 = Add(x=w358, y=w353) -> (x+y=w356:dbl)
            n211 = Add(x=w355, y=w354) -> (x+y=w351:dbl)
            n212 = local read "Y step size"() -> (w365:dbl)
            n213 = local read "X step size"() -> (w366:dbl)
            n214 = local read "state-queue"() -> (w370:T4)
            n215 = call "build-diode-scan-pts.vi"("Y step size"=w365, "X step size"=w366, "Y end"=w351, "Y start"=w352, "X end"=w356, "X start"=w357) -> ("y"=w368:dbl[], "x"=w369:dbl[])  [unwired: 4 in]
            n216 = for {
              tunnel: w369 -> [w384] mode=indexing
              tunnel: w368 -> [w383] mode=indexing
              shift-right: [w377] -> w367
              shift-left: w370 -> [w379]
              n217 = local read "next-state-cluster-const"() -> (w371:T1)
              n218 = Bundle By Name(cluster=w371, "next-state"="move", "bypass-confirm"=TRUE, "PDX"=w384, "PDY"=w383, "BarX"=93.0, "BarY"=20.0, "BMA"=45.0, "PDA"=181.0) -> (w378:T1)
              n219 = Bundle By Name(cluster=w371, "next-state"="log-pd3") -> (w372:T1)
              n220 = Build Array (concatenate)(w379, w378, w372) -> (w377:T4)
            }
            n221 = Array Size(array=w367) -> (size(s)=w364:i32)
            n222 = local write "queue-size"(w364) -> ()
          }
          frame "wait" {
            n223 = property on="start-msg" class="Str"("Visible"=TRUE) -> ()  [unwired: 2 in, 2 out]
            n224 = local write "start-msg"("\n\n\nProgram Delay Active\nfor User to Exit Laser Area" ("String")) -> ()
            n225 = Unbundle By Name(w388) -> ("PDX"=w389:dbl)
            n226 = Multiply(x=w389, y=1000.0) -> (x*y=w391:dbl)
            n227 = Wait (ms)(milliseconds to wait=w391) -> ()  [unwired: 1 out]
            n228 = local read "state-queue"() -> (w387:T4)
          }
          frame "nelder-mead" {
            w398 = ""
            n229 = property on="start-msg" class="Str"("Visible"=TRUE) -> ()  [unwired: 2 in, 2 out]
            n230 = local read "stage-error"() -> (w429:errorcluster)
            n231 = call "get-stage-positions.vi"("error in (no error)"=w429, "Cluster"=w414) -> ("error out"=w428:errorcluster, "stage positions"=w427:T2)  [unwired: 8 in]
            n232 = Unbundle By Name(w428) -> ("status"=w430:bool)
            n233 = local write "stage-error"(w428) -> ()
            n234 = local write "stage-stat"(w430) -> ()
            n235 = control-ref of="NM-pts-tested"() -> (w392:refnum<vi>)
            n236 = local read "meter-error"() -> (w434:errorcluster)
            n237 = local read "stage-error"() -> (w433:errorcluster)
            n238 = local read "meter-visa"() -> (w432:refnum<visa-resource-name>)
            n239 = local read "PD Values"() -> (w431:cluster{"PD1":dbl, "PD2":dbl, "PD3":dbl})
            n240 = local write "start-msg"("\n\n\n\nPerforming Automated\nAlignment.\n\nPlease Wait.\n" ("String")) -> ()
            n241 = Unbundle By Name(w427) -> ("PD Y"=w425:dbl, "PD X"=w426:dbl)
            n242 = Bundle By Name(cluster=T7 {"alpha"=1.0, "gamma"=2.0, "rho"=0.5, "sigma"=0.5, "simplex L"=0.5} ("NM-params"), "simplex L"=0.5, "sigma"=0.5) -> (w417:T7)
            n243 = call "auto_alignment-v3-1.vi"("meter-visa"=w432, "xStart"=w426, "yStart"=w425, "NM-params"=w417, "PD Values"=w431, "stage-refs"=w414, "NM-pts-tested"=w392, "meter-error"=w434, "stage-error"=w433, "bar-note"=w413, "meas#"=w412) -> ("Optimized Location"=→"Optimized Location":dbl[], "logfile-line-out"=w395:string, "meter-error-out"=w424:errorcluster, "run time (s)"=→"run time (min)":dbl, "stage-error-out"=w423:errorcluster)
            n244 = local write "meter-error"(w424) -> ()
            n245 = local write "stage-error"(w423) -> ()
            n246 = local write "keep-file"(TRUE ("keep-file")) -> ()
            n247 = local read "log-error"() -> (w410:errorcluster)
            n248 = local read "log-path"() -> (w411:path)
            n249 = Open/Create/Replace File(file path (use dialog)=w411, error in=w410, operation (0:open)=T6."open", access (0:read/write)=enum16{"read/write", "read-only", "write-only"}."read/write") -> (refnum out=w409:refnum<file>, error out=w405:errorcluster)  [unwired: 2 in, 1 out]
            n250 = Read from Text File(file (use dialog)=w409, error in=w405) -> (refnum out=w406:refnum<file>, text=w402:string, error out=w404:errorcluster)  [unwired: 2 in, 1 out]
            n251 = Equal?(x=w398, y=w402) -> (x = y?=w401:bool)
            n252 = Select(t="time\tpd1\tpd2\tpd3\tpd3/pd1\tpd2/pd1\tbx\tby\tpdx\tpdy\tpda\tbm\tbar-note\tmeas#\tpt#\n", s=w401, f=w398) -> (s? t:f=w399:string)
            n253 = Concatenate Strings(w399, w395) -> (w400:string)
            n254 = Write to Text File(file (use dialog)=w406, text=w400, error in=w404) -> (refnum out=w408:refnum<file>, error out=w407:errorcluster)  [unwired: 1 in, 1 out]
            n255 = Close File(refnum=w408, error in=w407) -> (error out=w403:errorcluster)  [unwired: 1 out]
            n256 = Unbundle By Name(w403) -> ()  [unwired: 1 out]
            n257 = local write "log-error"(w403) -> ()
            n258 = local read "state-queue"() -> (w435:T4)
          }
          frame "multi-trial" {
            n259 = local read "next-state-cluster-const"() -> (w436:T1)
            n260 = Initialize Array(w436, 0 ("dimension size")) -> (w444:T4)
            n261 = for {
              N: 20 -> [_]
              shift-right: [w465] -> w439
              shift-left: w444 -> [w466]
              tunnel: "PDX start" -> [w453]
              tunnel: "PDY start" -> [w449]
              w448 = 2.0
              n262 = Subtract(x=w449, y=w448) -> (x-y=w450:dbl)
              n263 = local read "bar-note"() -> (w446:u16)
              n264 = Add(x=w449, y=w448) -> (x+y=w451:dbl)
              n265 = Subtract(x=w453, y=w448) -> (x-y=w455:dbl)
              n266 = Add(x=w453, y=w448) -> (x+y=w454:dbl)
              n267 = call-poly <vilib>:"Random Number (Range).vi"("lower bound (0)"=w450, "upper bound (100)"=w451) -> ("number"=w447:dbl)  [unwired: 9 in]
              n268 = call-poly <vilib>:"Random Number (Range).vi"("lower bound (0)"=w455, "upper bound (100)"=w454) -> ("number"=w452:dbl)  [unwired: 9 in]
              n269 = local read "next-state-cluster-const"() -> (w462:T1)
              n270 = Bundle By Name(cluster=w462, "next-state"="move", "bypass-confirm"=TRUE, "PDX"=w452, "PDY"=w447, "BarX"=90.0, "BarY"=35.0, "BMA"=45.0, "PDA"=181.0, "bar-note"=w446) -> (w463:T1)
              n271 = Bundle By Name(cluster=w462, "next-state"="nelder-mead") -> (w464:T1)
              n272 = Build Array (concatenate)(w466, w463, w464) -> (w465:T4)
            }
            n273 = Bundle By Name(cluster=w436, "next-state"="diode-scan-center") -> (w437:T1)
            n274 = Build Array (concatenate)(w439, w437) -> (w438:T4)
          }
          frame "setup-IR" {
            # "Pure Beam (PB)\nPDX 266\nPDY 126\nBX 170\nBY 30\nBA 45\nPDA 180"
            # "IR1\nPDX 232\nPDY 119.5\nBX 85\nBY 20\nBA 17.148\nPDA 238\n\nIR2\nPDX 232\nPDY 119.5\nBX 85\nBY 15\nBA 17.148\nPDA 238\n\nIR3\nPDX 232\nPDY 119.5\nBX 85\nBY 32\nBA 17.148\nPDA 238"
            n275 = local read "state-queue"() -> (w481:T4)
            n276 = local read "next-state-cluster-const"() -> (w469:T1)
            n277 = Bundle By Name(cluster=w469, "next-state"="logfile-setup") -> (w470:T1)
            n278 = Build Array (concatenate)(w481, w470) -> (w471:T4)
            n279 = for {
              N: 10 -> [_]
              shift-right: [w575] -> w477
              shift-left: w471 -> [w583]
              shift-right: [w561] -> w478
              shift-left: u32 0 -> [w558]
              i -> [w574]
              # "PB"
              # "IR1"
              n280 = Multiply(x=0.1, y=w574) -> (x*y=w568:dbl)
              n281 = local read "next-state-cluster-const"() -> (w564:T1)
              n282 = Add(x=20.0, y=w568) -> (x+y=w554:dbl)
              n283 = Add(x=85.0, y=w568) -> (x+y=w555:dbl)
              n284 = Bundle By Name(cluster=w564, "next-state"="move", "bypass-confirm"=TRUE, "PDX"=223.0 ("BarX"), "PDY"=119.5 ("BarY"), "BarX"=w555, "BarY"=w554, "BMA"=17.148, "PDA"=238.0) -> (w579:T1)
              n285 = Bundle By Name(cluster=w564, "next-state"="move", "bypass-confirm"=TRUE, "PDX"=266.0 ("BarX"), "PDY"=126.0 ("BarY"), "BarX"=170.0 ("x"), "BarY"=30.0 ("x"), "BMA"=45.0, "PDA"=180.0) -> (w563:T1)
              n286 = Increment(x=w558) -> (x+1=w561:u32)
              n287 = Bundle By Name(cluster=w564, "next-state"="nelder-mead", "bar-note"=u8 1, "meas#"=w558) -> (w576:T1)
              n288 = Bundle By Name(cluster=w564, "next-state"="nelder-mead", "bar-note"=u8 0, "meas#"=w558) -> (w562:T1)
              n289 = Build Array (concatenate)(w583, w579, w576, w563, w562) -> (w575:T4)
            }
            n290 = for {
              N: 10 -> [_]
              shift-right: [w541] -> w475
              shift-left: w477 -> [w549]
              shift-right: [w527] -> w474
              shift-left: w478 -> [w524]
              i -> [w540]
              # "PB"
              # "IR1"
              n291 = Multiply(x=0.1, y=w540) -> (x*y=w534:dbl)
              n292 = local read "next-state-cluster-const"() -> (w530:T1)
              n293 = Add(x=20.0, y=w534) -> (x+y=w520:dbl)
              n294 = Add(x=85.0, y=w534) -> (x+y=w521:dbl)
              n295 = Bundle By Name(cluster=w530, "next-state"="move", "bypass-confirm"=TRUE, "PDX"=223.0 ("BarX"), "PDY"=119.5 ("BarY"), "BarX"=w521, "BarY"=w520, "BMA"=17.148, "PDA"=238.0) -> (w545:T1)
              n296 = Bundle By Name(cluster=w530, "next-state"="move", "bypass-confirm"=TRUE, "PDX"=266.0 ("BarX"), "PDY"=126.0 ("BarY"), "BarX"=170.0 ("x"), "BarY"=30.0 ("x"), "BMA"=45.0, "PDA"=180.0) -> (w529:T1)
              n297 = Increment(x=w524) -> (x+1=w527:u32)
              n298 = Bundle By Name(cluster=w530, "next-state"="nelder-mead", "bar-note"=u8 1, "meas#"=w524) -> (w542:T1)
              n299 = Bundle By Name(cluster=w530, "next-state"="nelder-mead", "bar-note"=u8 0, "meas#"=w524) -> (w528:T1)
              n300 = Build Array (concatenate)(w549, w545, w542, w529, w528) -> (w541:T4)
            }
            n301 = for {
              N: 10 -> [_]
              shift-right: [w507] -> w472
              shift-left: w475 -> [w515]
              shift-right: [w493] -> _
              shift-left: w474 -> [w490]
              i -> [w506]
              # "PB"
              # "IR1"
              n302 = Multiply(x=0.1, y=w506) -> (x*y=w500:dbl)
              n303 = local read "next-state-cluster-const"() -> (w496:T1)
              n304 = Add(x=20.0, y=w500) -> (x+y=w486:dbl)
              n305 = Add(x=85.0, y=w500) -> (x+y=w487:dbl)
              n306 = Bundle By Name(cluster=w496, "next-state"="move", "bypass-confirm"=TRUE, "PDX"=223.0 ("BarX"), "PDY"=119.5 ("BarY"), "BarX"=w487, "BarY"=w486, "BMA"=17.148, "PDA"=238.0) -> (w511:T1)
              n307 = Bundle By Name(cluster=w496, "next-state"="move", "bypass-confirm"=TRUE, "PDX"=266.0 ("BarX"), "PDY"=126.0 ("BarY"), "BarX"=170.0 ("x"), "BarY"=30.0 ("x"), "BMA"=45.0, "PDA"=180.0) -> (w495:T1)
              n308 = Increment(x=w490) -> (x+1=w493:u32)
              n309 = Bundle By Name(cluster=w496, "next-state"="nelder-mead", "bar-note"=u8 1, "meas#"=w490) -> (w508:T1)
              n310 = Bundle By Name(cluster=w496, "next-state"="nelder-mead", "bar-note"=u8 0, "meas#"=w490) -> (w494:T1)
              n311 = Build Array (concatenate)(w515, w511, w508, w495, w494) -> (w507:T4)
            }
          }
          frame "setup-BA" {
            # "Pure Beam (PB)\nPDX 266\nPDY 126\nBX 170\nBY 30\nBA 45\nPDA 180"
            # "BA1\nPDX 268\nPDY 126\nBX 229\nBY 30\nBA 45\nPDA 180\n\nBA2\nPDX 268\nPDY 126\nBX 229\nBY 15\nBA 45\nPDA 180\n\nBA3\nPDX 268\nPDY 126\nBX 229\nBY 20\nBA 45\nPDA 180"
            n312 = local read "state-queue"() -> (w597:T4)
            n313 = local read "next-state-cluster-const"() -> (w585:T1)
            n314 = Bundle By Name(cluster=w585, "next-state"="logfile-setup") -> (w586:T1)
            n315 = Build Array (concatenate)(w597, w586) -> (w587:T4)
            n316 = for {
              N: 10 -> [_]
              shift-right: [w691] -> w594
              shift-left: w587 -> [w699]
              shift-right: [w677] -> w592
              shift-left: u32 0 -> [w674]
              i -> [w690]
              # "PB"
              # "BA1"
              n317 = Multiply(x=0.1, y=w690) -> (x*y=w684:dbl)
              n318 = local read "next-state-cluster-const"() -> (w680:T1)
              n319 = Add(x=30.0, y=w684) -> (x+y=w670:dbl)
              n320 = Add(x=229.0, y=w684) -> (x+y=w671:dbl)
              n321 = Bundle By Name(cluster=w680, "next-state"="move", "bypass-confirm"=TRUE, "PDX"=268.0 ("BarX"), "PDY"=126.0 ("BarY"), "BarX"=w671, "BarY"=w670, "BMA"=45.0, "PDA"=180.0) -> (w695:T1)
              n322 = Bundle By Name(cluster=w680, "next-state"="move", "bypass-confirm"=TRUE, "PDX"=266.0 ("BarX"), "PDY"=126.0 ("BarY"), "BarX"=170.0 ("x"), "BarY"=30.0 ("x"), "BMA"=45.0, "PDA"=180.0) -> (w679:T1)
              n323 = Increment(x=w674) -> (x+1=w677:u32)
              n324 = Bundle By Name(cluster=w680, "next-state"="nelder-mead", "bar-note"=u8 2, "meas#"=w674) -> (w692:T1)
              n325 = Bundle By Name(cluster=w680, "next-state"="nelder-mead", "bar-note"=u8 0, "meas#"=w674) -> (w678:T1)
              n326 = Build Array (concatenate)(w699, w695, w692, w679, w678) -> (w691:T4)
            }
            n327 = for {
              N: 10 -> [_]
              shift-right: [w623] -> w593
              shift-left: w594 -> [w631]
              shift-right: [w609] -> w591
              shift-left: w592 -> [w606]
              i -> [w622]
              # "PB"
              # "BA2"
              n328 = Multiply(x=0.1, y=w622) -> (x*y=w616:dbl)
              n329 = local read "next-state-cluster-const"() -> (w612:T1)
              n330 = Add(x=15.0, y=w616) -> (x+y=w602:dbl)
              n331 = Add(x=229.0, y=w616) -> (x+y=w603:dbl)
              n332 = Bundle By Name(cluster=w612, "next-state"="move", "bypass-confirm"=TRUE, "PDX"=268.0 ("BarX"), "PDY"=126.0 ("BarY"), "BarX"=w603, "BarY"=w602, "BMA"=45.0, "PDA"=180.0) -> (w627:T1)
              n333 = Bundle By Name(cluster=w612, "next-state"="move", "bypass-confirm"=TRUE, "PDX"=266.0 ("BarX"), "PDY"=126.0 ("BarY"), "BarX"=170.0 ("x"), "BarY"=30.0 ("x"), "BMA"=45.0, "PDA"=180.0) -> (w611:T1)
              n334 = Increment(x=w606) -> (x+1=w609:u32)
              n335 = Bundle By Name(cluster=w612, "next-state"="nelder-mead", "bar-note"=u8 2, "meas#"=w606) -> (w624:T1)
              n336 = Bundle By Name(cluster=w612, "next-state"="nelder-mead", "bar-note"=u8 0, "meas#"=w606) -> (w610:T1)
              n337 = Build Array (concatenate)(w631, w627, w624, w611, w610) -> (w623:T4)
            }
            n338 = for {
              N: 10 -> [_]
              shift-right: [w657] -> w588
              shift-left: w593 -> [w665]
              shift-right: [w643] -> _
              shift-left: w591 -> [w640]
              i -> [w656]
              # "PB"
              # "BA3"
              n339 = Multiply(x=0.1, y=w656) -> (x*y=w650:dbl)
              n340 = local read "next-state-cluster-const"() -> (w646:T1)
              n341 = Add(x=20.0, y=w650) -> (x+y=w636:dbl)
              n342 = Add(x=229.0, y=w650) -> (x+y=w637:dbl)
              n343 = Bundle By Name(cluster=w646, "next-state"="move", "bypass-confirm"=TRUE, "PDX"=268.0 ("BarX"), "PDY"=126.0 ("BarY"), "BarX"=w637, "BarY"=w636, "BMA"=45.0, "PDA"=180.0) -> (w661:T1)
              n344 = Bundle By Name(cluster=w646, "next-state"="move", "bypass-confirm"=TRUE, "PDX"=266.0 ("BarX"), "PDY"=126.0 ("BarY"), "BarX"=170.0 ("x"), "BarY"=30.0 ("x"), "BMA"=45.0, "PDA"=180.0) -> (w645:T1)
              n345 = Increment(x=w640) -> (x+1=w643:u32)
              n346 = Bundle By Name(cluster=w646, "next-state"="nelder-mead", "bar-note"=u8 2, "meas#"=w640) -> (w658:T1)
              n347 = Bundle By Name(cluster=w646, "next-state"="nelder-mead", "bar-note"=u8 0, "meas#"=w640) -> (w644:T1)
              n348 = Build Array (concatenate)(w665, w661, w658, w645, w644) -> (w657:T4)
            }
          }
          frame "logfile-setup" {
            n349 = local read "log-path"() -> (w705:path)
            n350 = Path To String(path=w705) -> (string=w703:string)
            n351 = Concatenate Strings("Use logfile set at program start or start new file? \n\nLogfile set at start:\n", w703) -> (w702:string)
            n352 = Two Button Dialog(message=w702, 1:"Continue" ("F button name (\"Cancel\")"), 2:"Make New File" ("T button name (\"OK\")")) -> (T button?=w706:bool)
            n353 = case shown="True" w706 {
              frame False {
              }
              frame True {
                w710 = FALSE  # dev-mode
                n354 = call "log_file_setup.vi"("dev-mode"=w710) -> ("error out"=w708:errorcluster, "appended path"=w709:path)  [unwired: 8 in, 1 out]
                n355 = local write "log-path"(w709) -> ()
                n356 = local write "log-error"(w708) -> ()
              }
            }
            n357 = local read "state-queue"() -> (w707:T4)
          }
        }
        n358 = Subtract(x=w99, y=w98) -> (x-y=→"loop-rate":u32)
        n359 = Get Date/Time In Seconds() -> (seconds since 1Jan1904=w94:timestamp)
        n360 = Format Date/Time String(time format string (%c)="%Y-%m-%d %H:%M:%S", seconds (now)=w94) -> (date/time string=→"Current Time:":string)  [unwired: 1 in]
      }
    }
    frame #4 {
      # "close stages"
      n361 = local read "main-stage-refs"() -> (w711:T3)
      n362 = Unbundle By Name(w711) -> ("Bar X main"=w717:refnum<k24>, "Bar Y main"=w716:refnum<k24>, "PD X main"=w715:refnum<k24>, "PD Y main"=w714:refnum<k24>, "BMA main"=w713:refnum<k24>, "PDA main"=w712:refnum<k24>)
      n363 = invoke class="BenchtopStepperControl" method="CloseDevice"(reference=w713) -> (error out=w722:errorcluster)  [unwired: 2 in, 2 out]
      n364 = invoke class="BenchtopStepperControl" method="CloseDevice"(reference=w712) -> (error out=w723:errorcluster)  [unwired: 2 in, 2 out]
      n365 = invoke class="LongTravelStageControl" method="CloseDevice"(reference=w717) -> (error out=w718:errorcluster)  [unwired: 2 in, 2 out]
      n366 = invoke class="LongTravelStageControl" method="CloseDevice"(reference=w716) -> (error out=w719:errorcluster)  [unwired: 2 in, 2 out]
      n367 = invoke class="LongTravelStageControl" method="CloseDevice"(reference=w715) -> (error out=w720:errorcluster)  [unwired: 2 in, 2 out]
      n368 = invoke class="LongTravelStageControl" method="CloseDevice"(reference=w714) -> (error out=w721:errorcluster)  [unwired: 2 in, 2 out]
      n369 = local read "stage-error"() -> (w724:errorcluster)
      n370 = Merge Errors(w724, w718, w719, w720, w721, w722, w723) -> (w725:errorcluster)
      n371 = local write "stage-error"(w725) -> ()
    }
    frame #5 {
      # "Close connection to meter"
      n372 = local read "meter-error"() -> (w727:errorcluster)
      n373 = local read "meter-visa"() -> (w726:refnum<visa-resource-name>)
      n374 = call <instrlib>:"Close.vi"("error in (no error)"=w727, "VISA resource name"=w726) -> ("error out"=w728:errorcluster)  [unwired: 9 in]
      n375 = local write "meter-error"(w728) -> ()
    }
    frame #6 {
      # "Section deletes log file if nothing is written to it\nto prevent just a ton of empty files during development"
      n376 = local read "log-error"() -> (w731:errorcluster)
      n377 = local read "keep-file"() -> (w729:bool)
      n378 = local read "log-path"() -> (w730:path)
      n379 = case shown="False" w729 {
        tunnel: w731 -> [w734 w736]
        tunnel: [w735 w736] -> w732
        tunnel: w730 -> [w733 _]
        frame False {
          n380 = Delete(path (use dialog)=w733, error in=w734) -> (error out=w735:errorcluster)  [unwired: 3 in, 2 out]
        }
        frame True {
        }
      }
      n381 = local write "log-error"(w732) -> ()
    }
  }
